vi "W7XBolo2018.vi"(1 "FPGA VI Reference In":refnum<k20>) -> (0 "FPGA VI Reference Out":refnum<k20>)   [LabVIEW 2014]
uses:
  <vilib>/Platform/TimedLoop/XDataNode/timing_clust.ctl
  <vilib>/Platform/TimedLoop/XDataNode/nitl_modes.ctl
  <vilib>/Platform/TimedLoop/XDataNode/wakeup.ctl
  <vilib>/userdefined/High Color/nirio_resource_hc.ctl
  <vilib>/DAQmx/write.llb/DAQmx Write (Analog 1D DBL 1Chan NSamp).vi
  <vilib>/FPGAPlugInAG/PCI-7813R/niLvFpga_Open_PCI-7813R.vi
  <vilib>/Utility/error.llb/Error Cluster From Error Code.vi
  <vilib>/rvi/errors/niLvFpgaAdjustHostInterfaceError.vi
  <vilib>/rvi/interface/common/niFpgaWaitOnOcc.vi
  <vilib>/DAQmx/create/channels.llb/DAQmx Create Channel (AO-Voltage-Basic).vi
  <vilib>/DAQmx/configure/timing.llb/DAQmx Timing (Sample Clock).vi
  <vilib>/DAQmx/miscellaneous.llb/DAQmx Fill In Error Info.vi
  <vilib>/httpClient/POSTBuffer.vi
  <vilib>/FPGAPlugInAG/PCI-7813R/niLvFpga_Close_PCI-7813R.vi
  <vilib>/Utility/file.llb/Read From Spreadsheet File (DBL).vi
  <vilib>/Utility/file.llb/Read From Spreadsheet File (I64).vi
  <vilib>/Platform/TimedLoop/XDataNode/XDataNode.xnode
  <vilib>/rvi/interface/nirviOpenFPGA/nirviOpenFPGA.xnode
  FPGA Bitfiles/W7XBolo2017_FPGATarget_fmain2014_9xlV3GyHFfo.lvbitx
  f_main_2014.vi
  <vilib>/rvi/interface/nirviReadWriteControl/nirviReadWriteControl.xnode
  <vilib>/rvi/interface/nirviMethod/nirviMethod.xnode
  <vilib>/rvi/interface/nirviCloseFPGA/nirviCloseFPGA.xnode
  <vilib>/Platform/TimedLoop/XDataNode/XDNodeRunTimeDep.lvlib
  <vilib>/Analysis/NI_AALBase.lvlib
  <vilib>/httpClient/LabVIEWHTTPClient.lvlib
  <resource>/objmgr/daqmx.rc
  NiFpgaLv.dll
  <vilib>/FPGAPlugInAG/PCI-7813R/niLvFpga_AcknowledgeIrq_PCI-7813R.vi
  <vilib>/FPGAPlugInAG/PCI-7813R/niLvFpga_ConfigureFifo_PCI-7813R.vi
  <vilib>/rvi/errors/niLvFpgaMergeErrorWithErrorCode.vi
panel:
  out "Time until Acqusition":dbl(slide)=4294967295.0 scale=0.0..60.0
  out "start time":i64
  out "trigger time final":i64
  out "DAQ Timer":dbl
  in  "Tab Control 7":T1(tab)
  in  "FreqSelRing":u16(ring) items=["0.8 ms", "1.6 ms", "3.2 ms", "6.4 ms", "12.8 ms", "19.2 ms"]
  in  "SecondFilter":bool=TRUE
  out "SampleTime":sgl=0.0008
  in  "global or individual DAC settings for knob":bool caption="Range?"
  in  "DAC Range Setting":u8(knob)=3 scale=0.0..3.0
  out "No. of Samples\n[TOA / Sample Rate]":u32=10000
  out "Measured Time for DAQ [ms]\n\nApprox. ~ SampleTime * Samples":u32
  in  "?":bool=TRUE
  in  "DAC settings file location":path=path "C:/LABVIEW/BLV Philipp/LABVIEW/BLV/bolo_files/dac_settings.dat"
  in  "Time of Acqusition [s]":dbl=10.0
  out "predicted time [ms] to finalize DAQ":dbl
  in  "Read Channel Selection from file":bool=TRUE
  in  "Path to channel selection file":path=path "C:/LABVIEW/BLV Philipp/LABVIEW/BLV/bolo_files/short_channel_selection.dat"
  in  "Path to kbolott and volume data file":path=path "C:/LABVIEW/BLV Philipp/LABVIEW/BLV/bolo_files/kbolott_volume_all.dat"
  in  "Read geometry from file?":bool=TRUE
  in  "Trigger Source":i32(slide)=2 scale=0.0..3.0
  in  "Set Manual Time [ns], default updated last on 06/20/2018":i64=1529501124000000000
  out "Presamples \n(If -1, then no trigger detected)":i32
  out "DAQ wait time (should be = TWT":i32=-1
  out "Countdown Time":u32
  out "Calibration Time":u32
  out "Total wait time (TWT)\nTypically 59 s":u32
  in  "Pre-start time (ms) of DAQ \nTypically set to 1000 ms":i32=1000
  in  "Fixed T-60sec before T1 = T0":i32=60000
  in  "waiting time 'til trigger\npublished by CODAC":u32=10000
  out "Number of nanoseconds with offset to 1904":i64
  out "current epoch time timestamp":timestamp
  in  "Tau00":dbl[](array[numeric])=[0.11491729291343579, 0.11716798919571741, 0.11740631364396965, 0.11663726342199245, 0.41599980468961384, 0.11981011551839264, 0.11846429840933606, 0.11867732465684001, 0.1099546558688366, 0.11157519276959196, 0.10652596659944064, 0.11187533014192738, 0.11242534122168901, 0.11250590452650158, 0.11233958629056463, 0.11088956837703348, 0.11684290859752998, 0.11711408209103276, 0.11862962903855054, 0.11574688850921441, 0.11080958640139682, 0.11308007616237671, 0.11316833203019577, 0.11732662567656041, 0.11776955995449861, 0.11488434870753593, 0.11721346913661516, 0.11723600482803162, 0.1173219143188469, 0.11486538187917118, 0.1161354905419326, 0.11580597702447244, 0.11089805083278159, 0.10965173450878267, 0.10989266890532523, 0.11049724960692761, 0.11094253276914103, 0.1112015939579455, 0.11056511595580205, 0.11125203268352817, 0.10851766683731974, 0.10665739286095859, 0.10665088457538054, 0.10647759616581123, 0.10805487600009084, 0.10533289893772232, 0.10446227511758968, 0.10416638033440741, 0.11156846805821136, 0.11129308727212155, 0.11117840263008584, 0.1102971572868625, 0.10837301568677209, 0.11586325578254852, 0.11338638335503164, 0.11266837385466463, 0.11020464539493718, 0.11718312222258088, 0.11005940383900907, 0.11074035298635442, 0.11310264754168789, 0.11428021968521139, 0.10890693978140649, 0.11304857784773828, 0.11071164775178235, 0.10899043148625223, 0.1098152132889097, 0.11071094104034687, 0.10922727710545306, 0.11026461123495493, 0.10902110264823185, 0.1063818330991493, 0.1082901421909468, 0.10855104773097228, 0.10976304069098969, 0.1092806529611063, 0.10813898027014157, 0.10856892511543396, 0.10528805150138838, 0.10996755406311447, 0.11441717863822966, 0.11512938300201939, 0.11354812708860414, 0.11170183444428032, 0.10929951535815542, 0.10880924561891742, 0.11032002393110663, 0.12233406623444484, 0.10819046523889579, 0.10676534101945172, 0.11334069041654328, 0.11395839570756812, 0.10860855876008385, 0.11000092792604536, 0.11150855742531308, 0.11072296835591808, 0.11248944715419666, 0.11109385151927784, 0.10904702395407219, 0.0, 0.11012618939531567, 0.1101228599630128, 0.10901646637252452, 0.10848342666256441, 0.1118672405375629, 0.11165093132257785, 0.11030651312297526, 0.1105637825970819, 0.10972695234743621, 0.11008183794997571, 0.10869604711918752, 0.0, 0.10947241009391531, 0.5898071300815099, 0.41732939048318163, 0.0, 0.0, 0.0, 0.0, 0.0, 0.0, 0.0, 0.5051635137410128, 0.0, 0.0, 0.0, 0.4056247218989413, 0.0, 0.11491729291343579]
  in  "Kappa00":dbl[](array[numeric])=[0.0008402794220111138, 0.0008162628511746609, 0.0008306690902202418, 0.000803901120831155, 0.0003482758920990883, 0.0008106589659042871, 0.0008016286027972057, 0.000799559666964026, 0.0008329596140242245, 0.0008550459829924856, 0.0007662506038997399, 0.0008054791716010769, 0.0008538518247154832, 0.0008293547031323884, 0.0008561853513376051, 0.0008533408283799155, 0.0008374094293251158, 0.0008246891754373999, 0.0008094405414334474, 0.0008290847564626268, 0.00020601047667132065, 0.000800173048893566, 0.0007793179002779764, 0.0007971071724399289, 0.0007885266906587188, 0.0007777314742190596, 0.000805938950941268, 0.0007876903707101731, 0.0008486502743123638, 0.0008188176160358826, 0.0008275575494250777, 0.0008021526930523769, 0.0004219866202355569, 0.0008028836567896177, 0.0007965332650444257, 0.0007657694302588966, 0.0007891955147847732, 0.0007918255330716038, 0.0007896451983246505, 0.0007639621417921391, 0.0008241807402430576, 0.0008494655305824806, 0.0008513286284044697, 0.0008584599469876866, 0.0008065529851855167, 0.0008583681445476364, 0.0008848769105909991, 0.0008824761623272339, 0.0008739299904558458, 0.0008726933272884011, 0.0008591817798513973, 0.0008546408142867519, 0.0008814192063552359, 0.000837962132357275, 0.0008754373245495078, 0.0008659455513111399, 0.000875854800823488, 0.0008145627712648352, 0.000847096348180231, 0.0008354027185001123, 0.0008988684127044384, 0.0009087972104601418, 0.000872460372055295, 0.0008865774530667089, 0.0008205858447961992, 0.0008661153610700915, 0.0008514123741077071, 0.0008674455175914637, 0.0008535020874821334, 0.0008530135268333135, 0.0008817680910658127, 0.0008857682842425993, 0.0009014333315122717, 0.0009058705470039874, 0.0009451074888355545, 0.0008658347728111954, 0.0008865415114476586, 0.0009037142514292518, 0.0009300212486309693, 0.0009201252229947723, 0.0008662494433570838, 0.0008561155107896092, 0.0008934103962644251, 0.000843038472812381, 0.0008821165464311927, 0.0008725326170488139, 0.0008607956284658778, 0.0008692253024054895, 0.0007600922149492939, 0.0007595503979645458, 0.0008808740943017723, 0.0008427393057336779, 0.0008151549367042052, 0.0008178123459529788, 0.0008143006723436752, 0.0008042217964108747, 0.0007735257506859799, 0.0007705827889143488, 0.0007855750338204015, 1.5378016423296697e-10, 0.0007777843483157151, 0.0007914940873736198, 0.0007883969825026242, 0.000818379256343944, 0.0008183032224836934, 0.0008253700992517207, 0.0008193590844345892, 0.0008108478163956726, 0.0007992276276126246, 0.0007886605041422787, 0.000781928010070813, 1.3117348375603198e-11, 0.0007692233287415738, -6.433477601629483e-12, 5.840652071940865e-11, -5.095362431956802e-12, 1.483332911600832e-10, -2.3650890104320048e-11, 2.0638470359814695e-11, -4.2942497083098924e-12, -1.609109206826474e-13, -8.281241741308274e-13, -1.484842606490482e-11, 1.312154360785075e-10, -1.3280672580076002e-10, 3.875382814091509e-11, -5.840342459280051e-12, 1.6602972107316198e-05]
  in  "RB000":dbl[](array[numeric])=[962.4177063722611, 982.55505646202, 1001.4524254455091, 1013.2686972880372, 987.9006509030032, 991.6776299499904, 1028.1941896508492, 1025.4234890548287, 979.6474971153391, 974.5100933960157, 973.0002231971498, 981.3770747072988, 943.3083319407024, 941.9659261539757, 935.9901166328577, 922.8756359883505, 1000.2356401751263, 1016.4518014388639, 1008.5518682535671, 995.9759478197891, 1393.1164953762932, 1009.4128515400009, 1004.0036749391834, 998.4245511355359, 1013.969149931135, 1006.3653804065095, 999.1527693687324, 1010.8263977028598, 907.9396854856363, 919.914547854408, 928.8836112172035, 935.6473530653229, 1831.0832629084102, 903.0974305802013, 913.186368963444, 930.0383764679839, 876.4924197978996, 886.7670713082508, 894.536808158485, 915.0431333478505, 950.9758424469715, 947.5925766523108, 943.7054707777233, 932.0275841045941, 942.1982964674207, 920.3009912512268, 906.1613034702182, 900.8719996970515, 995.3340306419007, 1002.2623248554355, 1009.982778992568, 1020.4549365978846, 985.7853875544756, 1010.0388934379409, 924.365648284157, 938.198768243208, 984.5084426613569, 1028.1136001647244, 994.3062769668693, 996.1192994757585, 934.9355121674548, 939.7126408239549, 972.6026561318754, 952.3887606547273, 984.9574148687554, 938.8738492860468, 980.1140933255242, 976.5349653385726, 992.7415178653471, 992.5396366956102, 987.4159973831593, 984.3966487516718, 977.1474302625734, 949.6506551232892, 925.9244618646749, 977.9525359780853, 965.5702842228591, 958.1238603805732, 947.99064876123, 929.4112824181327, 921.0026412584975, 923.0539958218653, 922.9112208417712, 993.6091773425921, 967.4949115866236, 971.1288101242847, 976.32752644686, 1330.674292830122, 949.3495655938384, 944.3884832069355, 931.3665988355956, 938.4573966906173, 873.9327397917785, 861.7506061462778, 853.2628755931436, 852.3451337346856, 952.8804870925069, 966.9750479771292, 968.5993925762996, 0.0, 932.9605694732488, 935.3958729949309, 938.085486227425, 937.2411392500057, 848.2825097854029, 856.1379994596109, 865.233945109098, 882.1024138917886, 890.4810243739747, 897.2026495346195, 913.1867276731607, 0.0, 917.2859168494497, 0.0, 0.0, 0.0, 0.0, 0.0, 0.0, 0.0, 0.0, 0.0, 0.0, 0.0, 0.0, 0.0, 0.0, 0.0]
  in  "Switch to fixed \nCalibration Values":bool
  in  "Clear all Values \nfrom Beginning":bool
  in  "Cancel Button":bool
  out "Actual Depth":u32=256
  out "T-Start [for Display)\nShould be -1 [s]":sgl=-1.0
  in  "Trigger No Choice\nfrom MDS+ Website\n0 for old\n1 during OP":i32
  out "ScandID read/write error, late":errorcluster
  out "ScanID":u32
  in  "Tab Control":T2(tab)
  in  "Tab Control 4":enum32{"1 to 64", "65 to 128"}(tab)
  out "Raw 33-64":T3={"Channels 33 - 40"={"tstart"=-1.0, "FPGSampleTime"=0.0007999999797903001, array8x10000[80000 elements]}, "Channels 41 - 48"={"tstart"=-1.0, "FPGSampleTime"=0.0007999999797903001, array8x10000[80000 elements]}, "Channels 49 - 56"={"tstart"=-1.0, "FPGSampleTime"=0.0007999999797903001, array8x10000[80000 elements]}, "Channels 57 - 64"={"tstart"=-1.0, "FPGSampleTime"=0.0007999999797903001, array8x10000[80000 elements]}}
  out "Raw 1-32":T4={"Channels 1- 8"={"tstart"=-1.0, "FPGSampleTime"=0.0007999999797903001, array8x10000[80000 elements]}, "Channels 9 - 16"={"tstart"=-1.0, "FPGSampleTime"=0.0007999999797903001, array8x10000[80000 elements]}, "Channels 17 - 24"={"tstart"=-1.0, "FPGSampleTime"=0.0007999999797903001, array8x10000[80000 elements]}, "Channels 25 - 32"={"tstart"=-1.0, "FPGSampleTime"=0.0007999999797903001, array8x10000[80000 elements]}}
  out "Raw 97 - 128":T5
  out "Raw 65 - 97":T6={"Channels 65 - 71"={"tstart"=-1.0, "FPGSampleTime"=0.0007999999797903001, array8x10000[80000 elements]}, "Channels 73 - 80"={"tstart"=0.0, "FPGSampleTime"=0.0, []}, "Channels 81 - 88"={"tstart"=0.0, "FPGSampleTime"=0.0, []}, "Channels 89- 96"={"tstart"=0.0, "FPGSampleTime"=0.0, []}}
  out "RawArray":sgl[][](array[numeric])
  in  "Tab Control 6":enum32{"1 to 64", "65 to 128"}(tab)=enum."65 to 128"
  out "Pow 33-64":T3
  out "Pow 1-32":T4={"Channels 1- 8"={"tstart"=-1.0, "FPGSampleTime"=0.0007999999797903001, array8x10000[80000 elements]}, "Channels 9 - 16"={"tstart"=-1.0, "FPGSampleTime"=0.0007999999797903001, array8x10000[80000 elements]}, "Channels 17 - 24"={"tstart"=0.0, "FPGSampleTime"=0.0, []}, "Channels 25 - 32"={"tstart"=0.0, "FPGSampleTime"=0.0, []}}
  out "Pow 97 - 128":T5
  out "Pow 65 - 96":T6={"Channels 65 - 71"={"tstart"=-1.0, "FPGSampleTime"=0.0007999999797903001, array8x10000[80000 elements]}, "Channels 73 - 80"={"tstart"=0.0, "FPGSampleTime"=0.0, []}, "Channels 81 - 88"={"tstart"=0.0, "FPGSampleTime"=0.0, []}, "Channels 89- 96"={"tstart"=0.0, "FPGSampleTime"=0.0, []}}
  out "PowerArray":sgl[][](array[numeric])
  out "real time P_rad plot":cluster{i32, "element":dbl, "element":dbl}[](graph)
  out "Channel Selection\nfrom input?":bool
  out "DAC settings":i64[](array[numeric])=[3, 3, 3, 3, 3, 3, 3, 3, 3, 3, 3, 3, 3, 3, 3, 3, 3, 3, 3, 3, 3, 3, 3, 3, 3, 3, 3, 3, 3, 3, 3, 3, 3, 3, 3, 3, 3, 3, 3, 3, 3, 3, 3, 3, 3, 3, 3, 3, 3, 3, 3, 3, 3, 3, 3, 3, 3, 3, 3, 3, 3, 3, 3, 3, 3, 3, 3, 3, 3, 3, 3, 3, 3, 3, 3, 3, 3, 3, 3, 3, 3, 3, 3, 3, 3, 3, 3, 3, 3, 3, 3, 3, 3, 3, 3, 3, 3, 3, 3, 3, 3, 3, 3, 3, 3, 3, 3, 3, 3, 3, 3, 3, 3, 3, 3, 3, 3, 3, 3, 3, 3, 3, 3, 3, 3, 3, 0, 0]
  out "size(s)":i32
  out "Take file for DAC?":bool
  out "full DAC\nfile input":i64[][](array[numeric])=[[3], [3], [3], [3], [3], [3], [3], [3], [3], [3], [3], [3], [3], [3], [3], [3], [3], [3], [3], [3], [3], [3], [3], [3], [3], [3], [3], [3], [3], [3], [3], [3], [3], [3], [3], [3], [3], [3], [3], [3], [3], [3], [3], [3], [3], [3], [3], [3], [3], [3], [3], [3], [3], [3], [3], [3], [3], [3], [3], [3], [3], [3], [3], [3], [3], [3], [3], [3], [3], [3], [3], [3], [3], [3], [3], [3], [3], [3], [3], [3], [3], [3], [3], [3], [3], [3], [3], [3], [3], [3], [3], [3], [3], [3], [3], [3], [3], [3], [3], [3], [3], [3], [3], [3], [3], [3], [3], [3], [3], [3], [3], [3], [3], [3], [3], [3], [3], [3], [3], [3], [3], [3], [3], [3], [3], [3]]
  in  "input DAC settings":i64[](array[numeric])=[3, 3, 3, 3, 3, 3, 3, 3, 3, 3, 3, 3, 3, 3, 3, 3, 3, 3, 3, 3, 3, 3, 3, 3, 3, 3, 3, 3, 3, 3, 3, 3, 3, 3, 3, 3, 3, 3, 3, 3, 3, 3, 3, 3, 3, 3, 3, 3, 3, 3, 3, 3, 3, 3, 3, 3, 3, 3, 3, 3, 3, 3, 3, 3, 3, 3, 3, 3, 3, 3, 3, 3, 3, 3, 3, 3, 3, 3, 3, 3, 3, 3, 3, 3, 3, 3, 3, 3, 3, 3, 3, 3, 3, 3, 3, 3, 3, 3, 3, 3, 3, 3, 3, 3, 3, 3, 3, 3, 3, 3, 3, 3, 3, 3, 3, 3, 3, 3, 3, 3, 3, 3, 3, 3, 3, 3, 0, 0]
  out "Take Input for DAC?":bool
  out "kbolott_and_volume":dbl[][](array[numeric])
  out "final channel\nselection size":i32
  out "final channel selection":i64[][](array[numeric])=[[0], [1], [2], [3], [4], [5], [6], [7], [8], [9], [10], [11], [12], [13], [14], [15], [16], [17], [18], [19], [20], [21], [22], [23], [24], [25], [26], [27], [28], [29], [30], [31]]
  in  "channel selection input":i32[][](array[numeric])=[[1]]
  out "file import":i64[][](array[numeric])
  in  "maximum voltage @ 10MW\nP_rad estimate":dbl=10.0 format="%#_13g"
  out "number of samples per iteration":dbl
  out "number of samples written on channel":u32
  in  "rate of voltage sampling":dbl=100000.0 format="%#_13g"
  in  "RegenMode":i32(ring)=10158 items=["Allow Regeneration"=10097, "Do Not Allow Regeneration"=10158]
  in  "sample mode":i32(ring)=10123 items=["Finite Samples"=10178, "Continuous Samples"=10123, "Hardware Timed Single Point"=12522]
  in  "Stop Voltage Output":bool
  out "current P_rad sample [MW]":dbl format="%#_13g"
  out "final P_rad":dbl[](array[numeric])
  out "av power array":dbl[](array[numeric])
  out "P_rad analog output error source":string
  in  "DAQmx Physical Channel\nP_rad estimate":tag="Dev1/ao0"
  out "nominator":dbl
  out "number of samples \nwritten per channel":u32
  in  "selected channel for output via second analog channel":i32
  in  "estimated floating voltage":dbl format="%#_13g"
  out "estimated voltage @ 10 MW":dbl
  out "voltage factor":dbl
  in  "DAQmx Physical Channel\nsingle channel":tag="Dev1/ao1"
  in  "maximum voltage @ 10MW single channel":dbl=10.0 format="%#_13g"
  out "single channel output error source":string
  out "current single channel voltage":dbl format="%#_13g"
  out "single channel voltage array":dbl[](array[numeric])
  out "P_rad output\nvoltage":dbl
  out "single channel voltage output [MW]":dbl
  in  "voltage fac":dbl=10000.0
  out "RangeIndex":u8[](array[numeric])
  out "DACbits 2":u16[](array[numeric])
  out "x*2^n":sgl[](array[numeric])
  in  "Tab Control 2":T7(tab)
  out "Offset 1-32":T4
  out "Offset 33-64":T3
  out "Offset 65 - 96":T6
  out "Offset 97 - 128":T5
  out "Mean (mV)":dbl[](array[numeric]) format="%10.6f"
  out "Peak to Peak \n      (microV)":dbl[](array[numeric]) format="%10.6f"
  out "StandardDeviation\n        (microV)":dbl[](array[numeric]) format="%10.7f"
  out "Offset (V)":dbl[](array[numeric])
  out "RefStatus 65-96":bool[](array[boolean])
  out "RefStatus 33-64":bool[](array[boolean])
  out "RefStatus 1-32":bool[](array[boolean])
  out "RefStatus 97-128":bool[](array[boolean])
  out "MessStatus 1-32":bool[](array[boolean])
  out "MessStatus 33-64":bool[](array[boolean])
  out "MessStatus 97-128":bool[](array[boolean])
  out "MessStatus 65-96":bool[](array[boolean])
  in  "Tab Control 5":T8(tab)
  out "MessCal 17-32":T9
  out "MessCal 1-16":T10
  out "MessCal 49 - 64":T11
  out "MessCal 33 - 49":T12
  out "MessCal 81 - 96":T13
  out "MessCal 65 - 80":T14
  out "MessCal 113 - 128":T15
  out "MessCal 97 - 112":T16
  out "TauM":dbl[](array[numeric]) format="%10.4f"
  out "KappaM":dbl[](array[numeric]) format="%10.4e"
  out "RMESS":dbl[](array[numeric])
  out "RawScal":dbl[](array[numeric])
  out "ScalPower":dbl[](array[numeric])
  out "Tau":dbl[](array[numeric])
  out "F_ch":dbl[](array[numeric])
  out "tau_fact":dbl[](array[numeric])
  in  "Tab Control 3":T8(tab)=enum."97 to 128"
  out "RefCal 17-32":T9
  out "RefCal 1-16":T10
  out "RefCal 49 - 64":T11
  out "RefCal 33 - 48":T12
  out "RefCal 65 - 80":T14
  out "RefCal 81 - 96":T13
  out "RefCal 113 - 128":T15
  out "RefCal 97 - 112":T16
  out "TauR":dbl[](array[numeric]) caption="TauM" format="%10.4f"
  out "KappaR":dbl[](array[numeric]) format="%10.4e"
  out "RREF":dbl[](array[numeric])
  out "BoloCalibRefFoilFit data error":errorcluster
  out "BoloCalibRefFoilCurrent data error":errorcluster
  out "fpga_reference\nOpen error out":errorcluster
  out "Timed Out 2":bool
  out "Fehler":bool
  out "Fehler READ U+P":bool
  out "FilterTimeOut":bool
  out "result":bool
  out "error out Cal":errorcluster
  out "headers chanDesc":string="HTTP/1.1 201 Created\r\nServer: Apache-Coyote/1.1\r\nLocation: http://archive-webapi.ipp-hgw.mpg.de/Test/raw/W7X/QSB_Bolometry/File_PARLOG/\r\nContent-Type: text/plain\r\nTransfer-Encoding: chunked\r\nDate: Wed, 15 Jul 2015 13:52:20 GMT\r\n\r\n"
  out "body chanDesc":string="Test/raw/W7X/QSB_Bolometry/File_PARLOG/ created."
  out "parms error out":errorcluster
  out "error after hReadDMA":errorcluster
  out "ScandID read/write error, early":errorcluster
  out "ScanID 2":u32
  out "BoloCalibMeasFoilFit data error":errorcluster
  out "BoloSignal data error":errorcluster
  out "BoloCalibMeasFoilCurrent\ndata error":errorcluster
  out "rRes parlog error":errorcluster
  out "rKappa parlog error":errorcluster
  out "mTau parlog error":errorcluster
  out "offset parlog error":errorcluster
  out "mRes parlog error":errorcluster
  out "mKappa parlog error":errorcluster
  out "rTau parlog error":errorcluster
  out "loop error":errorcluster
  out "sampling error":errorcluster
  out "voltage sampling error":T17
  in  "SubVI Test\nwith RAND array and\ntime measurement":bool
  out "random array sub":dbl[](array[numeric])
  out "random array main":dbl[](array[numeric])
  out "sample array":i32[](array[numeric])
  out "subvi cycle #":dbl
  out "subvi timing":dbl
  out "pick-up cycle":i32
  out "total\ntime":dbl
  out "timing average":dbl format="%.2f"
  out "rand array sub display":dbl[](array[numeric])
  out "rand plot sub":cluster{i32, "element":dbl}[](graph)
  out "cycle #":i32
  out "rand plot main":cluster{i32, "element":dbl}[](graph)
  out "empty write array":dbl[](array[numeric])
  out "Nsample array":i32[](array[numeric])
  in  "stop":bool
  out "Acquired Samples:":u32(slide)=4294967295 scale=-1.0..10000.0
  out "state":string="Wait for Start"
  # "largest offset ~ 40 mV\n-- 40 mV should work --\n-- 80 mV safe setting --"
  # "Sample Rate Settings"
  # "FilterSelection"
  # "put time stamp of now as\nPOSIX time in [ns] as trigger"
  # "Set manual time\n[epoch time, ns since 01.01.1970]"
  # "Get last trigger from \nhttp://sv-coda-wsvc-3/last_trigger"
  # "Get UTC Time not working"
  # "WENDELSTEIN - 7-X Bolometer DAQ System [mail at: pih@ipp.mpg.de]"
  # "ver 2018"
  # "If individual Range DAC Setting is selected, \nthe gain Range is loaded from following file:"
  # "DAC Range shown for check:"
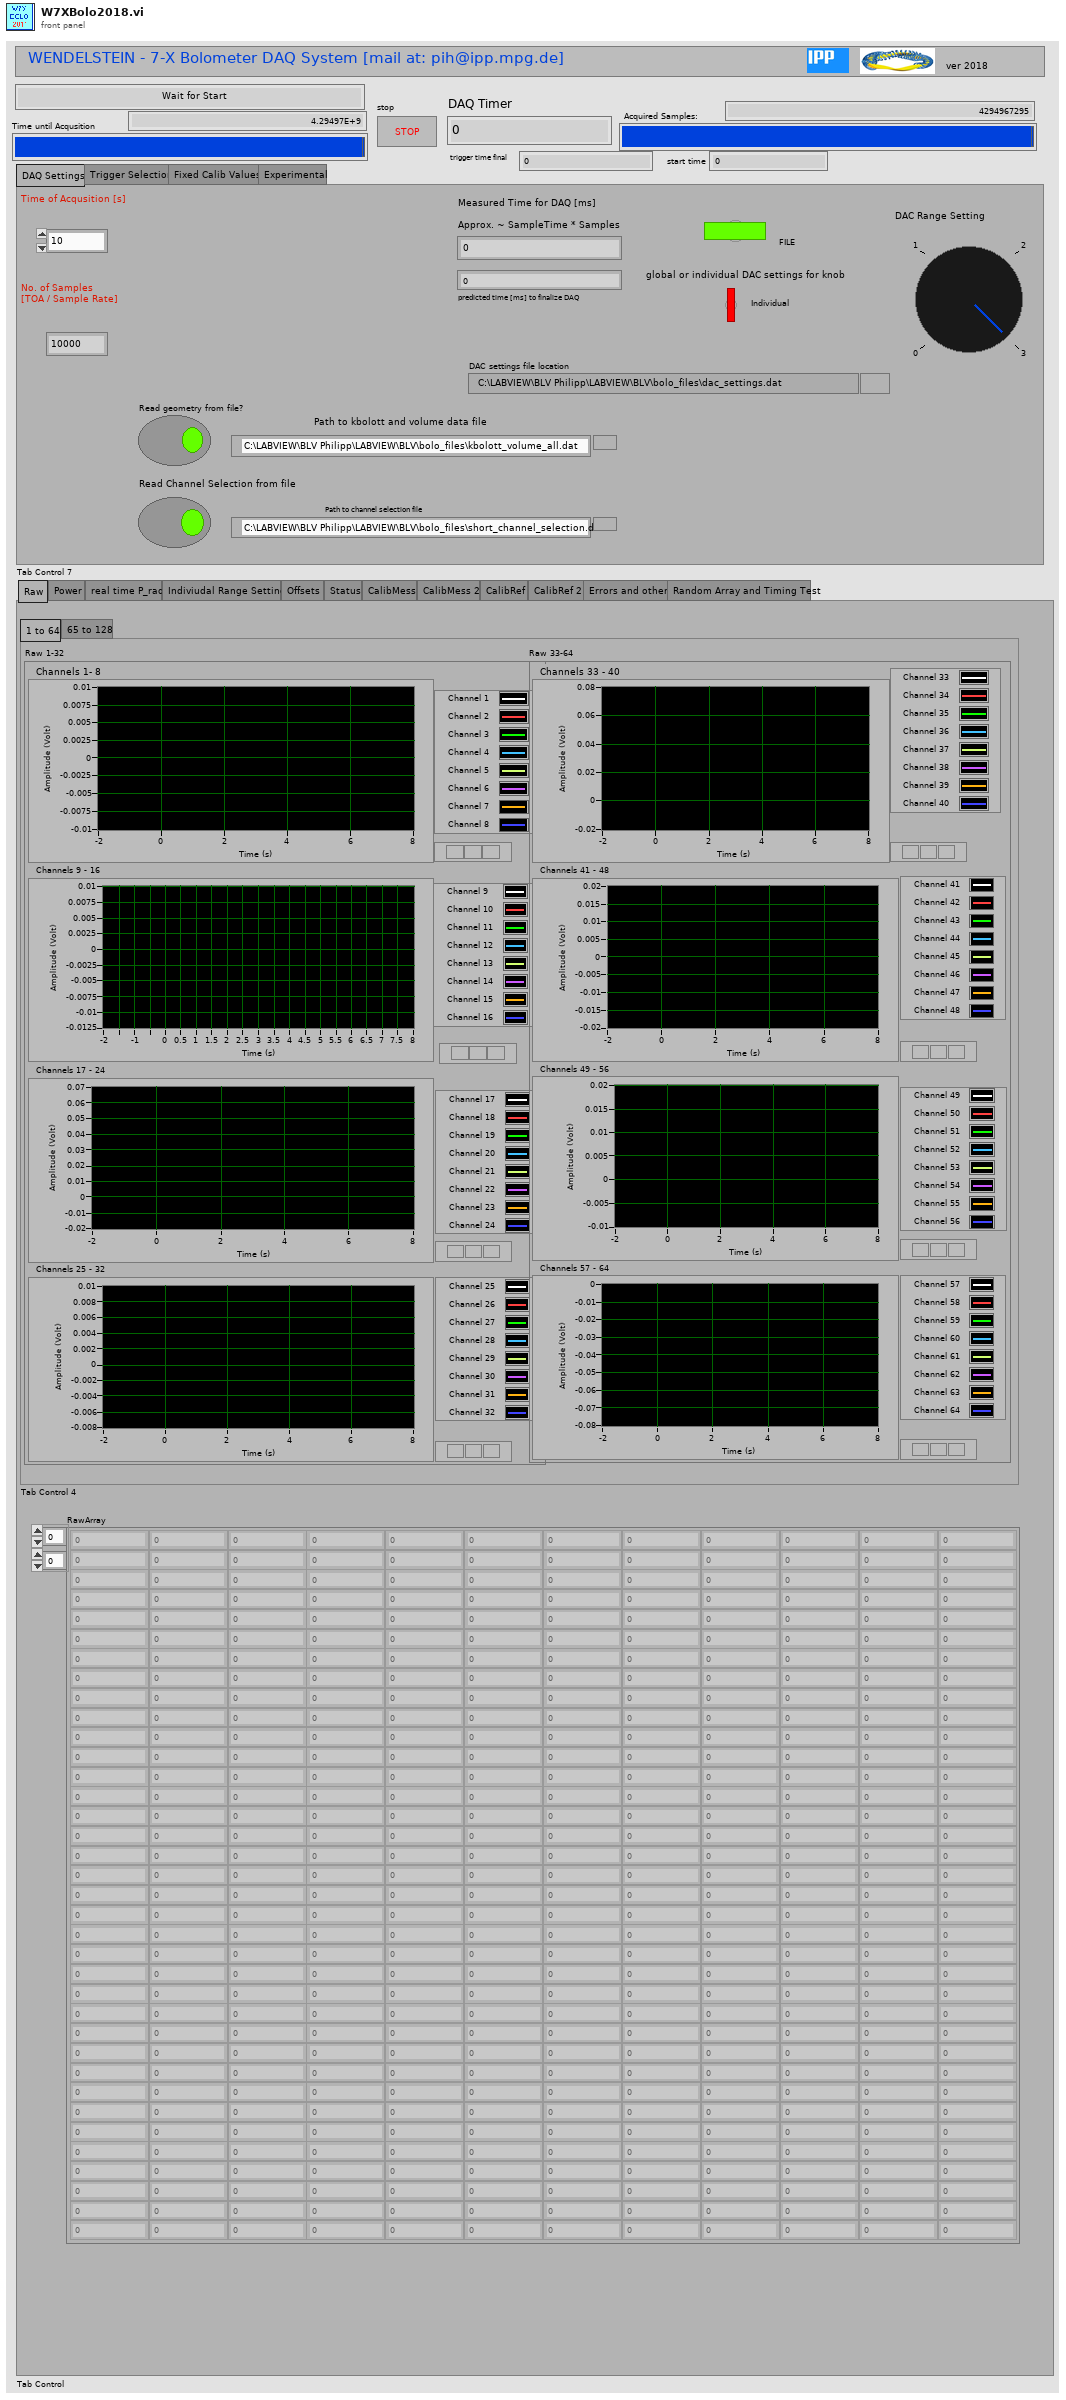
[diagram p1: front panel]
types:
  T1 = enum32{"DAQ Settings", "Trigger Selection", "Fixed Calib Values", "Experimental"}
  T2 = enum32{"Raw", "Power", "real time P_rad", "Indiviudal Range Settings", "Offsets", "Status", "CalibMess", "CalibMess 2", "CalibRef", "CalibRef 2", "Errors and others", "Random Array and Timing Test"}
  T3 = cluster{"Channels 33 - 40":cluster{"tstart":dbl, "FPGSampleTime":dbl, dbl[][]}, "Channels 41 - 48":cluster{"tstart":dbl, "FPGSampleTime":dbl, dbl[][]}, "Channels 49 - 56":cluster{"tstart":dbl, "FPGSampleTime":dbl, dbl[][]}, "Channels 57 - 64":cluster{"tstart":dbl, "FPGSampleTime":dbl, dbl[][]}}
  T4 = cluster{"Channels 1- 8":cluster{"tstart":dbl, "FPGSampleTime":dbl, dbl[][]}, "Channels 9 - 16":cluster{"tstart":dbl, "FPGSampleTime":dbl, dbl[][]}, "Channels 17 - 24":cluster{"tstart":dbl, "FPGSampleTime":dbl, dbl[][]}, "Channels 25 - 32":cluster{"tstart":dbl, "FPGSampleTime":dbl, dbl[][]}}
  T5 = cluster{"Channels 97 - 104":cluster{"tstart":dbl, "FPGSampleTime":dbl, dbl[][]}, "Channels 105 - 112":cluster{"tstart":dbl, "FPGSampleTime":dbl, dbl[][]}, "Channels 113 - 120":cluster{"tstart":dbl, "FPGSampleTime":dbl, dbl[][]}, "Channels 121 - 128":cluster{"tstart":dbl, "FPGSampleTime":dbl, dbl[][]}}
  T6 = cluster{"Channels 65 - 71":cluster{"tstart":dbl, "FPGSampleTime":dbl, dbl[][]}, "Channels 73 - 80":cluster{"tstart":dbl, "FPGSampleTime":dbl, dbl[][]}, "Channels 81 - 88":cluster{"tstart":dbl, "FPGSampleTime":dbl, dbl[][]}, "Channels 89- 96":cluster{"tstart":dbl, "FPGSampleTime":dbl, dbl[][]}}
  T7 = enum32{"1 to 32", "33 to 64", "65 to 96", "97 to128"}
  T8 = enum32{"1 to 32", "33 to 64", "65 to 96", "97 to 128"}
  T9 = cluster{"Channels 17 - 20":cluster{"tstart":sgl, "dt":sgl, "OutArray":dbl[][]}, "Channels 21 - 24":cluster{"tstart":sgl, "dt":sgl, "OutArray":dbl[][]}, "Channels 25 - 28":cluster{"tstart":sgl, "dt":sgl, "OutArray":dbl[][]}, "Channels 29 - 32":cluster{"tstart":sgl, "dt":sgl, "OutArray":dbl[][]}}
  T10 = cluster{"Channels 1- 4":cluster{"tstart":sgl, "dt":sgl, "OutArray":dbl[][]}, "Channels 5 - 8":cluster{"tstart":sgl, "dt":sgl, "OutArray":dbl[][]}, "Channels 9 - 12":cluster{"tstart":sgl, "dt":sgl, "OutArray":dbl[][]}, "Channels 13 - 16":cluster{"tstart":sgl, "dt":sgl, "OutArray":dbl[][]}}
  T11 = cluster{"Channels 49 - 52":cluster{"tstart":sgl, "dt":sgl, "OutArray":dbl[][]}, "Channels 53 - 56":cluster{"tstart":sgl, "dt":sgl, "OutArray":dbl[][]}, "Channels 57 - 60":cluster{"tstart":sgl, "dt":sgl, "OutArray":dbl[][]}, "Channels 61 - 64":cluster{"tstart":sgl, "dt":sgl, "OutArray":dbl[][]}}
  T12 = cluster{"Channels 33 - 36":cluster{"tstart":sgl, "dt":sgl, "OutArray":dbl[][]}, "Channels 37 - 40":cluster{"tstart":sgl, "dt":sgl, "OutArray":dbl[][]}, "Channels 41 - 44":cluster{"tstart":sgl, "dt":sgl, "OutArray":dbl[][]}, "Channels 45 - 48":cluster{"tstart":sgl, "dt":sgl, "OutArray":dbl[][]}}
  T13 = cluster{"Channels 81 - 84":cluster{"tstart":sgl, "dt":sgl, "OutArray":dbl[][]}, "Channels 85 - 88":cluster{"tstart":sgl, "dt":sgl, "OutArray":dbl[][]}, "Channels 89 - 92":cluster{"tstart":sgl, "dt":sgl, "OutArray":dbl[][]}, "Channels 93 - 96":cluster{"tstart":sgl, "dt":sgl, "OutArray":dbl[][]}}
  T14 = cluster{"Channels 65 - 68":cluster{"tstart":sgl, "dt":sgl, "OutArray":dbl[][]}, "Channels 69 - 72":cluster{"tstart":sgl, "dt":sgl, "OutArray":dbl[][]}, "Channels 73 - 76":cluster{"tstart":sgl, "dt":sgl, "OutArray":dbl[][]}, "Channels 77 - 80":cluster{"tstart":sgl, "dt":sgl, "OutArray":dbl[][]}}
  T15 = cluster{"Channels 113 - 116":cluster{"tstart":sgl, "dt":sgl, "OutArray":dbl[][]}, "Channels 117 - 120":cluster{"tstart":sgl, "dt":sgl, "OutArray":dbl[][]}, "Channels 121 - 124":cluster{"tstart":sgl, "dt":sgl, "OutArray":dbl[][]}, "Channels 125 - 128":cluster{"tstart":sgl, "dt":sgl, "OutArray":dbl[][]}}
  T16 = cluster{"Channels 97 - 100":cluster{"tstart":sgl, "dt":sgl, "OutArray":dbl[][]}, "Channels 101 - 104":cluster{"tstart":sgl, "dt":sgl, "OutArray":dbl[][]}, "Channels 104 - 108":cluster{"tstart":sgl, "dt":sgl, "OutArray":dbl[][]}, "Channels 109 - 112":cluster{"tstart":sgl, "dt":sgl, "OutArray":dbl[][]}}
  T17 = cluster{"error out":errorcluster, "error out":errorcluster}
  T18 = cluster{"Nchannel":i16, "ADCbits":i16, "BridgeVoltage (V)":sgl, "ExptSampleFrequency (Hz)":sgl, "CalibSampleFrequency (Hz)":sgl, "CalStep1 (V)":string, "CalStep2 (V)":string, "detector":string}[]
  T19 = cluster{"chanDescs":cluster{"name":string, "active":i32}[]}[]
  T20 = cluster{"tstart":sgl, "dt":sgl, "OutArray":dbl[][]}
  T21 = cluster{"Channels 9 - 12":cluster{"tstart":sgl, "dt":sgl, "OutArray":dbl[][]}, "Channels 9 - 12":cluster{"tstart":sgl, "dt":sgl, "OutArray":dbl[][]}, "Channels 9 - 12":cluster{"tstart":sgl, "dt":sgl, "OutArray":dbl[][]}, "Channels 9 - 12":cluster{"tstart":sgl, "dt":sgl, "OutArray":dbl[][]}}
  T22 = typedef "nirio_resource_hc.ctl" = tag
  T23 = typedef "XDNodeRunTimeDep.lvlib/timing_clust.ctl" = cluster{"Expected End [f-1]":u64, "Actual End [f-1]":u64, "Finished Late? [f-1]":bool, "Expected End [i-1]":u64, "Actual End [i-1]":u64, "Finished Late? [i-1]":bool, "Expected Start [i]":u64, "Actual Start [i]":u64, "Expected Start [f]":u64, "Actual Start [f]":u64, "Source Name":string, "Structure Name":string, "Period":i64, "Deadline":i64, "Offset":i64, "Start":i64, "Priority":i32, "Timeout":i32, "Mode":T24, "Wakeup Reason":T25, "Error":errorcluster, "Source Type":string, "Secondary Source Type":string, "Global End Time":u64, "Global Start Time":u64, "Frame Duration":u64, "Iteration Duration":u64, "Assigned CPU":i32, "I/O Scan Engine Mode":u32}
  T24 = typedef "XDNodeRunTimeDep.lvlib/nitl_modes.ctl" = enum32{"No Change", "Process missed periods, maintain original phase", "Discard missed periods, maintain original phase", "Process missed periods, ignore original phase", "Discard missed periods, ignore original phase"}
  T25 = typedef "XDNodeRunTimeDep.lvlib/wakeup.ctl" = enum32{"Normal", "Aborted", "Asynchronous wakeup", "Timing source error", "Timed loop error", "Timeout"}
  T26 = cluster{"Channels 33 - 40":cluster{"tstart":dbl, "FPGSampleTime":dbl, dbl[][]}, "Channels 41 - 48":cluster{"tstart":dbl, "FPGSampleTime":dbl, dbl[][]}, "Channels 49 - 56":cluster{"tstart":dbl, "FPGSampleTime":dbl, dbl[][]}, "Channels 57 - 58":cluster{"tstart":dbl, "FPGSampleTime":dbl, dbl[][]}}
  T27 = cluster{"Channels 1- 8":cluster{"tstart":sgl, "dt":sgl, "OutArray":dbl[][]}, "Channels 9 - 16":cluster{"tstart":sgl, "dt":sgl, "OutArray":dbl[][]}, "Channels 17 - 24":cluster{"tstart":sgl, "dt":sgl, "OutArray":dbl[][]}, "Channels 25 - 32":cluster{"tstart":sgl, "dt":sgl, "OutArray":dbl[][]}}
  T28 = cluster{"Channels 33 - 40":cluster{"tstart":sgl, "dt":sgl, "OutArray":dbl[][]}, "Channels 41 - 48":cluster{"tstart":sgl, "dt":sgl, "OutArray":dbl[][]}, "Channels 49 - 56":cluster{"tstart":sgl, "dt":sgl, "OutArray":dbl[][]}, "Channels 57 - 58":cluster{"tstart":sgl, "dt":sgl, "OutArray":dbl[][]}}
  T29 = typedef "LabVIEWHTTPClient.lvlib/ClientHandle.ctl" = refnum<k1>
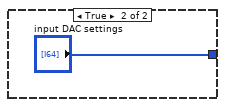
[diagram p4: hidden frame]
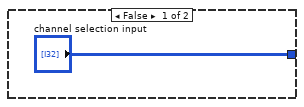
[diagram p6: hidden frame]
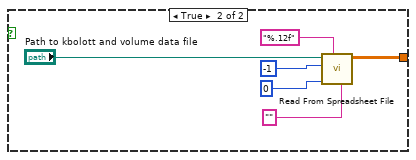
[diagram p8: hidden frame]
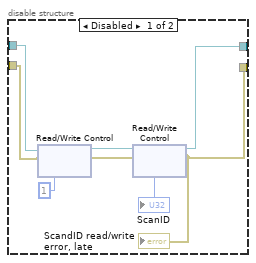
[diagram p15: hidden frame]
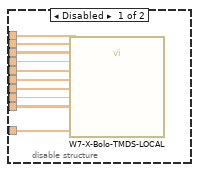
[diagram p18: hidden frame]
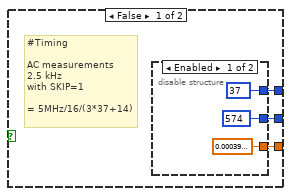
[diagram p19: hidden frame]
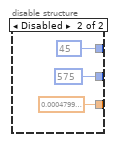
[diagram p20: hidden frame]
diagram:
  w28 = i64 -1  # Time Array needs to be positive!
  w47 = i64 -1000000000  # Ns per Sec
  w83 = 1 ("sampleCount")
  w84 = 1 ("sampleCount")
  w87 = "s"  # Unit
  w108 = "V"  # Unit
  w112 = "A"  # Unit
  w24 = "A"  # Unit
  w116 = "A"  # Unit
  w123 = 1 ("sampleCount")
  w125 = 1 ("sampleCount")
  w127 = 1 ("sampleCount")
  w82 = 1 ("sampleCount")
  w53 = 1 ("sampleCount")
  w133 = "Float"  # datatype
  w103 = "mV"  # Unit
  w105 = "Offset"  # label
  w139 = "Float"  # datatype
  w100 = "W"  # Unit
  w102 = "RKappa"  # label
  w141 = "Float"  # datatype
  w97 = "Ohms"  # Unit
  w99 = "RRes"  # label
  w143 = "Float"  # datatype
  w94 = "s"  # Unit
  w96 = "RTau"  # label
  w145 = "Float"  # datatype
  w91 = "W"  # Unit
  w93 = "MKappa"  # label
  w147 = "Float"  # datatype
  w90 = "Ohms"  # Unit
  w89 = "MRes"  # label
  w149 = "Float"  # datatype
  w86 = "MTau"  # label
  w54 = 10000 ("dimension size")
  w157 = 10000 ("sampleCount")
  w159 = "Float"  # datatype
  w118 = "A"  # Unit
  w120 = "BoloCalibRefFoilFit"  # label
  w160 = 10000 ("sampleCount")
  w162 = "Float"  # datatype
  w114 = "BoloCalibRefFoilCurrent"  # label
  w163 = 10000 ("sampleCount")
  w165 = "Float"  # datatype
  w23 = "BoloCalibMeasFoilFit"  # label
  w166 = 10000 ("sampleCount")
  w168 = "Float"  # datatype
  w110 = "BoloCalibMeasFoilCurrent"  # label
  w169 = "Float"  # datatype
  w107 = "BoloSignal"  # label
  # "Negative Sample Time [ns]"
  # "Time array for Bolo Signal"
  # "No of Samples DAQ"
  # "Time array for Bolo Signal"
  # "+ wait Time"
  # "-800000ns for 0.8ms"
  # "Negative Sample Time [ns]"
  # "Here Changed Names"
  # "Time Stamp for JSON Files"
  # "Sample rate for Calibration Arrays\n should be hardwired to calirbation settings"
  # "Sample Rate in [ns]"
  # "Calculated Start Time [ns]"
  # "NSample"
  # "10000"
  # "Initialize Array:\nDimesions Size = NSamples"
  # "Pulselength fixed for 0.4ms sample time and 10000 samples"
  # "NSamples * SampleTime = PulseLength"
  # "Data here is incorrect as well=!"
  # "Sample Time [s]\ncalculated to \nSample Time [ns]"
  # "Creating virtual Time Stamp\nfor Shot and for Calibration (Hardwired to 10000 samples)\nShot is depending on set sample rate"
  # "Index von dem Sample\nals der Trigger empfangen wurde"
  # "T1 Trigger\nkommt hier"
  # "A=> Internal full scale calibration\n8=> Internal zero scale calibration\nC=> System Zero scale Calibration\n2=> Continuous conversion\n\n5V reference\n80 mV scale\nChannel 1 input (voltage at bridge)\nMaster clock disable\n\np.15 7730 manual"
  # "AC 1.25 kHz Frequenz\nSKIP=0"
  n1 = call <vilib>:"High Resolution Relative Seconds.vi"() -> ("relative seconds"=w15:dbl)
  n2 = flat-sequence {
    tunnel: [w226] -> w72
    tunnel: ["FPGA VI Reference In"] -> w75
    tunnel: [w227] -> w16
    tunnel: w72 -> [w227]
    frame #0 {
      n3 = Tick Count (ms)() -> (millisecond timer value=w226:u32)
    }
    frame #1 {
      n4 = case shown="True" "Clear all Values \nfrom Beginning" {
        frame False {
        }
        frame True {
          n5 = flat-sequence {
            frame #0 {
              w232 = bool[] [] ("MessStatus 1-32")
              w231 = dbl[] [] ("Kappa00")
              w234 = T20 {"tstart"=0.0, "dt"=0.0, "OutArray"=[]} ("Channels 9 - 12")
              # "Clear Graphs"
              n6 = local write "RREF"(w231) -> ()
              n7 = local write "Kappa00"(w231) -> ()
              n8 = local write "TauR"(w231) -> ()
              n9 = local write "Tau00"(w231) -> ()
              n10 = local write "RB000"(w231) -> ()
              n11 = local write "RefStatus 97-128"(w232) -> ()
              n12 = local write "RefStatus 1-32"(w232) -> ()
              n13 = local write "RefStatus 33-64"(w232) -> ()
              n14 = local write "RefStatus 65-96"(w232) -> ()
              n15 = local write "KappaR"(w231) -> ()
              n16 = local write "RMESS"(w231) -> ()
              n17 = local write "MessStatus 1-32"(w232) -> ()
              n18 = local write "MessStatus 33-64"(w232) -> ()
              n19 = local write "MessStatus 65-96"(w232) -> ()
              n20 = local write "MessStatus 97-128"(w232) -> ()
              n21 = local write "KappaM"(w231) -> ()
              n22 = local write "DACbits 2"(w231) -> ()
              n23 = local write "TauM"(w231) -> ()
              n24 = Bundle("Channels 9 - 12"=w234, "Channels 9 - 12"=w234, "Channels 9 - 12"=w234, "Channels 9 - 12"=w234) -> (w233:T21)  [unwired: 1 in]
              n25 = local write "Raw 1-32"(w233) -> ()
              n26 = local write "Raw 33-64"(w233) -> ()
              n27 = local write "Pow 1-32"(w233) -> ()
              n28 = local write "Pow 33-64"(w233) -> ()
              n29 = local write "RangeIndex"(w231) -> ()
              n30 = local write "Mean (mV)"(w231) -> ()
              n31 = local write "Peak to Peak \n      (microV)"(w231) -> ()
              n32 = local write "StandardDeviation\n        (microV)"(w231) -> ()
              n33 = local write "Acquired Samples:"(0) -> ()
              n34 = local write "Raw 65 - 97"(w233) -> ()
              n35 = local write "Raw 97 - 128"(w233) -> ()
              n36 = local write "Offset 1-32"(w233) -> ()
              n37 = local write "Offset 33-64"(w233) -> ()
              n38 = local write "Offset 65 - 96"(w233) -> ()
              n39 = local write "Offset 97 - 128"(w233) -> ()
              n40 = local write "RefCal 1-16"(w233) -> ()
              n41 = local write "RefCal 113 - 128"(w233) -> ()
              n42 = local write "RefCal 17-32"(w233) -> ()
              n43 = local write "RefCal 33 - 48"(w233) -> ()
              n44 = local write "RefCal 49 - 64"(w233) -> ()
              n45 = local write "RefCal 65 - 80"(w233) -> ()
              n46 = local write "RefCal 81 - 96"(w233) -> ()
              n47 = local write "RefCal 97 - 112"(w233) -> ()
              n48 = local write "Pow 65 - 96"(w233) -> ()
              n49 = local write "Pow 97 - 128"(w233) -> ()
              n50 = local write "MessCal 1-16"(w233) -> ()
              n51 = local write "MessCal 113 - 128"(w233) -> ()
              n52 = local write "MessCal 17-32"(w233) -> ()
              n53 = local write "MessCal 33 - 49"(w233) -> ()
              n54 = local write "MessCal 49 - 64"(w233) -> ()
              n55 = local write "MessCal 65 - 80"(w233) -> ()
              n56 = local write "MessCal 81 - 96"(w233) -> ()
              n57 = local write "MessCal 97 - 112"(w233) -> ()
            }
          }
        }
      }
    }
  }
  n58 = disable-structure shown="Disabled" {
    frame Disabled {
      n59 = case shown="True" "SubVI Test\nwith RAND array and\ntime measurement" {
        frame False {
        }
        frame True {
          n60 = flat-sequence {
            tunnel: [w240] -> w237
            tunnel: [w239] -> w236
            tunnel: w237 -> [w255]
            tunnel: w236 -> [w249]
            frame #0 {
              w239 = 1000 ("x")
              n61 = Initialize Array(0, w239) -> (w244:i32[])
              n62 = for {
                N: w239 -> [_]
                shift-right: [w245] -> w240
                shift-left: w244 -> [w247]
                i -> [w246]
                n63 = Replace Array Subset(array=w247, new element=w246, index=w246) -> (w245:i32[])
              }
              "sample array" <- w240
              n64 = local write "state"("pre-occupying test arrays" ("state")) -> ()
              n65 = Initialize Array(0.0 ("element"), w239) -> (w238:dbl[])
              "random array main" <- w238
              "random array sub" <- w238
              n66 = local write "random array main"(w238) -> ()
              n67 = local write "random array sub"(w238) -> ()
            }
            frame #1 {
              # "testing for array output"
              n68 = call <vilib>:"High Resolution Relative Seconds.vi"() -> ("relative seconds"=w251:dbl)
              n69 = control-ref of="rand array sub display"() -> (w253:refnum<vi>)
              n70 = local read "No. of Samples\n[TOA / Sample Rate]"() -> (w248:u32)
              n71 = for {
                N: w248 -> [_]
                i -> [w261]
                n72 = local read "av power array"() -> (w265:dbl[])
                n73 = local read "final P_rad"() -> (w262:dbl[])
                n74 = Random Number (0-1)() -> (number: 0 to 1=w264:dbl)
                n75 = Replace Array Subset(array=w265, new element=w264, index=w261) -> (w263:dbl[])
                n76 = Random Number (0-1)() -> (number: 0 to 1=w260:dbl)
                n77 = Replace Array Subset(array=w262, new element=w260, index=w261) -> (w259:dbl[])
                n78 = local write "av power array"(w263) -> ()
                n79 = local write "final P_rad"(w259) -> ()
                n80 = Wait Until Next ms Multiple(millisecond multiple=u32 50) -> ()  [unwired: 1 out]
              }
              n81 = control-ref of="subvi cycle #"() -> (w250:refnum<vi>)
              n82 = control-ref of="subvi timing"() -> (w252:refnum<vi>)
              n83 = for {
                N: w249 -> [_]
                tunnel: w255 -> [w278]
                i -> [w279]
                n84 = local read "random array main"() -> (w277:dbl[])
                n85 = Wait Until Next ms Multiple(millisecond multiple=10) -> ()  [unwired: 1 out]
                n86 = Random Number (0-1)() -> (number: 0 to 1=w281:dbl)
                n87 = Replace Array Subset(array=w277, new element=w281, index=w279) -> (w276:dbl[])
                n88 = Build Cluster Array(w278, w276) -> (→"rand plot main":cluster{i32, "element":dbl}[])
                n89 = local write "random array main"(w276) -> ()
                "cycle #" <- w279
              }
              n90 = local read "random array sub"() -> (w254:dbl[])
              n91 = control-ref of="rand plot sub"() -> (w256:refnum<vi>)
              n92 = local write "state"("subvi and real time plot" ("state")) -> ()
              n93 = call "test.vi"("length"=w249, "subvi cycle"=w250, "sample array"=w255, "rand array sub"=w254, "subvi timing"=w252, "Graph Refnum"=w256, "start time"=w251, "rand array sub refnum"=w253) -> ()  [unwired: 4 in]
              n94 = while {
                tunnel: w251 -> [w273]
                tunnel: w249 -> [w267]
                i -> [w269]
                stop <- w274 stop-if-true
                n95 = Multiply(x=w267, y=10) -> (x*y=w268:i32)
                n96 = call <vilib>:"High Resolution Relative Seconds.vi"() -> ("relative seconds"=w272:dbl)
                n97 = Greater?(x=w268, y=w269) -> (0:w274:bool)
                n98 = Subtract(x=w272, y=w273) -> (x-y=w271:dbl)
                "total\ntime" <- w271
                n99 = Divide(x=w271, y=w269) -> (x/y=→"timing average":dbl)
                n100 = Wait Until Next ms Multiple(millisecond multiple=1) -> ()  [unwired: 1 out]
                "pick-up cycle" <- w269
              }
            }
          }
        }
      }
    }
    frame Enabled {
    }
  }
  n101 = Not A Number/Path/Refnum?(number/path/refnum=w75) -> (NaN/Path/Refnum?=w17:bool)
  n102 = case shown="True" w17 {
    tunnel: [w283 w285] -> w12
    tunnel: [_ w284] -> w13
    tunnel: w75 -> [w283 _]
    frame False {
    }
    frame True {
      n103 = xnode "Open FPGA VI Reference"("resource name"=T22 "RIO0") -> ("FPGA VI Reference Out"=w285:refnum<k20>, "error out"=w284:errorcluster)  [unwired: 1 in]
    }
  }
  "fpga_reference\nOpen error out" <- w13
  n104 = disable-structure shown="Enabled" {
    disable-tunnel: w15 -> [w287 _]
    frame Enabled {
      n105 = while {
        tunnel: w287 -> [w295]
        i -> [w305]
        stop <- w306 stop-if-true
        n106 = local read "Fixed T-60sec before T1 = T0"() -> (w291:i32)
        n107 = local read "Pre-start time (ms) of DAQ \nTypically set to 1000 ms"() -> (w301:i32)
        n108 = Divide(x=w291, y=1000) -> (x/y=w289:dbl)
        n109 = Divide(x=w301, y=1000) -> (x/y=w298:dbl)
        n110 = To Quad Integer(1:w298) -> (0:w299:i64)
        n111 = To Quad Integer(1:w289) -> (0:w288:i64)
        n112 = Subtract(x=w288, y=w299) -> (x-y=w296:i64)
        n113 = call <vilib>:"High Resolution Relative Seconds.vi"() -> ("relative seconds"=w293:dbl)
        n114 = To Double Precision Float(number=w296) -> (double precision float=w297:dbl)
        n115 = Add(x=w295, y=w297) -> (x+y=w294:dbl)
        n116 = Subtract(x=w294, y=w293) -> (x-y=→"Time until Acqusition":dbl)
        n117 = Get Date/Time In Seconds() -> (seconds since 1Jan1904=w312:timestamp)
        "current epoch time timestamp" <- w312
        n118 = To Quad Integer(1:w312) -> (0:w314:i64)
        n119 = Subtract(x=w314, y=2082844800) -> (x-y=w310:i64)
        n120 = Multiply(x=1000000000, y=w310) -> (x*y=w302:i64)
        "Number of nanoseconds with offset to 1904" <- w302
        n121 = Wait Until Next ms Multiple(millisecond multiple=1) -> ()  [unwired: 1 out]
        n122 = local read "state"() -> (w307:string)
        n123 = Equal?(x="Acquiring Data...", y=w307) -> (x = y?=w306:bool)
        n124 = Equal?(x=w305, y=0) -> (x = y?=w303:bool)
        n125 = case shown="True" w303 {
          tunnel: w302 -> [_ w315]
          frame False {
          }
          frame True {
            n126 = local write "start time"(w315) -> ()
            "start time" <- w315
          }
        }
      }
    }
    frame Disabled {
    }
  }
  n127 = disable-structure shown="Enabled" {
    frame Enabled {
      n128 = case shown="False" "Read geometry from file?" {
        tunnel: [w318 w319] -> w316
        frame False {
          n129 = call "load_kbolott_volume.vi"() -> ("output"=w318:dbl[][])
        }
        frame True {
          n130 = call-poly <vilib>:"Read From Spreadsheet File.vi"("delimiter (\\t)"="" ("delimiter (\\t)"), "format (%.3f)"="%.12f", "max characters/row  (no limit:0)"=0, "number of rows (all:-1)"=-1, "file path (dialog if empty)"="Path to kbolott and volume data file") -> ("all rows"=w319:dbl[][])  [unwired: 2 in, 4 out]
        }
      }
      "kbolott_and_volume" <- w316
      n131 = local write "kbolott_and_volume"(w316) -> ()
    }
    frame Disabled {
    }
  }
  n132 = disable-structure shown="Enabled" {
    frame Enabled {
      n133 = Not(x="Read Channel Selection from file") -> (.not. x?=→"Channel Selection\nfrom input?":bool)
      n134 = case shown="True" "Read Channel Selection from file" {
        tunnel: ["channel selection input" w332] -> w328
        frame False {
        }
        frame True {
          n135 = call-poly <vilib>:"Read From Spreadsheet File.vi"("delimiter (\\t)"="\t" ("delimiter (\\t)"), "format (%d)"="%d", "max characters/row  (no limit:0)"=0, "start of read offset (chars.:0)"=0, "number of rows (all:-1)"=-1, "file path (dialog if empty)"="Path to channel selection file") -> ("all rows"=w332:i64[][])  [unwired: 1 in, 4 out]
          "file import" <- w332
        }
      }
      "final channel selection" <- w328
      n136 = Array Size(array=w328) -> (size(s)=w327:i32[])
      n137 = local write "final channel selection"(w328) -> ()
      n138 = Index Array(array=w327, index=0) -> (element=→"final channel\nselection size":i32)
    }
    frame Disabled {
    }
  }
  n139 = disable-structure shown="Enabled" {
    frame Enabled {
      n140 = Not(x="?") -> (.not. x?=w342:bool)
      "Take Input for DAC?" <- w342
      n141 = case shown="False" w342 {
        tunnel: "DAC settings file location" -> [w350 _]
        tunnel: [w344 "input DAC settings"] -> w339
        frame False {
          n142 = call-poly <vilib>:"Read From Spreadsheet File.vi"("format (%d)"="%d", "max characters/row  (no limit:0)"=58, "number of rows (all:-1)"=-1, "file path (dialog if empty)"=w350) -> ("all rows"=w345:i64[][])  [unwired: 3 in, 4 out]
          "full DAC\nfile input" <- w345
          n143 = Reshape Array(w345, 128 ("dimension size")) -> (w344:i64[])
        }
        frame True {
        }
      }
      "DAC settings" <- w339
      n144 = local write "input DAC settings"(w339) -> ()
      n145 = Array Size(array=w339) -> (size(s)=→"size(s)":i32)
      "Take file for DAC?" <- "?"
    }
    frame Disabled {
    }
  }
  n146 = flat-sequence {
    tunnel: "Cancel" ("name (unnamed)") -> [w361]
    tunnel: "Transferred1" ("name (unnamed)") -> [w360]
    tunnel: u32 0 -> [w359]
    tunnel: FALSE -> [w358]
    tunnel: [w357] -> w216
    tunnel: [w356] -> w215
    tunnel: [w355] -> w214
    tunnel: [w354] -> w213
    tunnel: [u32 0] -> w78
    frame #0 {
      n147 = local write "stop"(FALSE ("stop")) -> ()
      n148 = RT FIFO Create(0:w360, 1:w359) -> (8:w354:refnum<k33>, 11:w355:errorcluster)  [unwired: 2 in, 5 out]
      n149 = RT FIFO Create(0:w361, 1:w358) -> (8:w357:refnum<k33>, 11:w356:errorcluster)  [unwired: 3 in, 4 out]
    }
  }
  n150 = xnode "Read/Write Control"("FPGA VI Reference In"=w12, "error in"=w13, "cancel"=TRUE ("clrFifo"), "Test"=FALSE) -> ("FPGA VI Reference Out"=w225:refnum<k20>, "error out"=w224:errorcluster)
  n151 = flat-sequence {
    tunnel: w225 -> [w368]
    tunnel: w224 -> [w367]
    tunnel: [w366] -> w223
    tunnel: [w365] -> w222
    frame #0 {
      n152 = Wait (ms)(milliseconds to wait=u32 100) -> ()  [unwired: 1 out]
      n153 = xnode "Invoke Method"("FPGA VI Reference In"=w368, "error in"=w367, "IRQ Number(s)"=i32[] [0, 1, 2, 3]) -> ("FPGA VI Reference Out"=w366:refnum<k20>, "error out"=w365:errorcluster)
      "state" <- "Start (100 ms)" ("state")
    }
  }
  n154 = node-c288() -> (w208:T23)  [unwired: 1 in, 4 out]
  n155 = timed-loop {
    tunnel: w216 -> [w379]
    tunnel: w215 -> [w378]
    tunnel: w214 -> [w377]
    tunnel: w213 -> [w376]
    tunnel: [w375] -> w210
    tunnel: [w374] -> w209
    tunnel: [w373] -> w212
    tunnel: [w372] -> w211
    timing: w208 -> [_]
    timing-out: [_] -> w207
    shift-right: [w369] -> _
    shift-left: w78 -> [w370]
    stop <- "stop" stop-if-true
    n156 = RT FIFO Read(0:w376, 1:w370, 3:w377) -> (8:w373:refnum<k33>, 9:w369:u32, 11:w372:errorcluster)  [unwired: 3 out]
    n157 = RT FIFO Write(0:w379, 1:"Cancel Button", 3:w378) -> (8:w375:refnum<k33>, 11:w374:errorcluster)  [unwired: 1 in, 3 out]
    "Acquired Samples:" <- w370
  }
  n158 = flat-sequence {
    tunnel: w222 -> [w384]
    tunnel: [w383] -> w204
    tunnel: w223 -> [w385]
    tunnel: [w386] -> w186
    frame #0 {
      n159 = local write "state"("Reset" ("state")) -> ()
      n160 = call "hReset2014.vi"("error in"=w384, "FPGA VI Reference In"=w385) -> ("error out"=w383:errorcluster, "FPGA VI Reference Out"=w386:refnum<k20>)  [unwired: 4 in]
    }
  }
  n161 = node-c288(w207) -> (→"loop error":errorcluster)  [unwired: 6 out]
  n162 = call "hFilterReg2014.vi"("error in"=w204, "Filter Modus"=u16 61 ("t"), "Frequenz"=u8 79 ("AC 1kHz Frequenz\nSKIP=0"), "FPGA VI Reference In"=w186) -> ("error out"=w189:errorcluster, "Timed Out"=w198:bool, "FPGA VI Reference Out"=w188:refnum<k20>)  [unwired: 1 in]
  "FilterTimeOut" <- w198
  n163 = call "hModeReg2014.vi"("error in"=w189, "Mode"=u16 41144, "FPGA VI Reference In"=w188) -> ("error out"=w192:errorcluster, "Timeout"=w202:bool, "FPGA VI Reference Out"=w195:refnum<k20>)  [unwired: 2 in]
  n164 = call "hModeReg2014.vi"("error in"=w192, "Mode"=u16 32952, "FPGA VI Reference In"=w195) -> ("error out"=w191:errorcluster, "Timeout"=w203:bool, "FPGA VI Reference Out"=w194:refnum<k20>)  [unwired: 2 in]
  n165 = flat-sequence {
    tunnel: w212 -> [w392]
    tunnel: w211 -> [w391]
    tunnel: w210 -> [w390]
    tunnel: w209 -> [w389]
    frame #0 {
      n166 = RT FIFO Delete(0:w392, 3:w391) -> ()  [unwired: 1 in, 1 out]
      n167 = RT FIFO Delete(0:w390, 3:w389) -> ()  [unwired: 1 in, 1 out]
      n168 = local write "stop"(FALSE ("stop")) -> ()
    }
  }
  n169 = call "hModeReg2014.vi"("error in"=w191, "Mode"=u16 8376, "FPGA VI Reference In"=w194) -> ("error out"=w200:errorcluster, "Timeout"=w201:bool, "FPGA VI Reference Out"=w199:refnum<k20>)  [unwired: 2 in]
  n170 = Compound Arithmetic op=OR(w202, w203, w201, w198) -> (w187:bool)
  "result" <- w187
  n171 = case shown="False" w187 {
    tunnel: [w456 w1095] -> w73
    tunnel: [w455 w1094] -> w221
    tunnel: w199 -> [w611 w1095]
    tunnel: w200 -> [w610 w1094]
    tunnel: [w474 _] -> w1
    tunnel: [w510 _] -> w155
    tunnel: [w505 _] -> w156
    tunnel: [w501 _] -> w153
    tunnel: [w498 _] -> w154
    tunnel: [w453 _] -> w76
    tunnel: [w496 _] -> w138
    tunnel: [w495 _] -> w77
    tunnel: [w494 _] -> w137
    tunnel: [w493 _] -> w136
    tunnel: [w472 _] -> w135
    tunnel: [w476 _] -> w29
    tunnel: w16 -> [w447 _]
    tunnel: [w446 _] -> w48
    tunnel: [w414 _] -> _
    frame False {
      w516 = 2000
      w527 = u8 125  # Frequenz
      w570 = 0.0008 ("FPGSampleTime")
      w565 = 0.0
      w436 = 40.0  # Rcable
      w605 = 10.0  # Rload
      w625 = sgl 0.0004  # dt
      w626 = sgl 0.0  # tstart
      w629 = sgl 0.0004  # dt
      w630 = sgl 0.0  # tstart
      w634 = sgl 80.0 ("Scale(mV)")
      # "Offset Shift manually disabled because not need for low power discharges"
      # "Local TDMS Data Storage"
      # "Absolute Timer [ms] (Now)\n-\nAbsolute Timer [ms] (At Start)\n=\nTime need until start of DAQ"
      # "Startzeit - 14 s"
      # "old time from OP1"
      # "Store raw data"
      # "#Timing \n\nAC measurements\n2.083 kHz\nwith SKIP=1 \n\n= 5MHz/16/(3*45+15)"
      # "#Offset measurement"
      # "#Offset applied"
      # "#Range for measurements"
      # "A=> Internal full scale calibration\n8=> Internal zero scale calibration\nC=> System Zero scale Calibration\n2=> Continuous conversion\n\n2.5V reference\n80 mV scale\nChannel 2 input (voltage at shunt)\nMaster clock disable\n\np.15 7730 manual"
      n172 = flat-sequence {
        tunnel: [w762] -> w451
        tunnel: [w761] -> w450
        tunnel: w611 -> [w765]
        tunnel: w610 -> [w764]
        tunnel: w516 -> [w770]
        tunnel: [w769] -> w518
        tunnel: w451 -> [w772]
        tunnel: w450 -> [w771]
        tunnel: [w768] -> w517
        tunnel: [w786] -> w689
        tunnel: [w785] -> w688
        tunnel: [w784] -> w437
        tunnel: w516 -> [w782]
        tunnel: w518 -> [w779]
        tunnel: w517 -> [w780]
        frame #0 {
          n173 = call "Wait3"("Count(mSec)"=u32 3000) -> ()  [unwired: 1 out]
          n174 = call "hComRegStart2013.vi"("error in"=w764, "FPGA VI Reference In"=w765) -> ("error out"=w761:errorcluster, "Timed Out"=→"Timed Out 2":bool, "FPGA VI Reference Out"=w762:refnum<k20>)  [unwired: 3 in]
        }
        frame #1 {
          n175 = local write "state"("SyncRun (1000 ms)" ("state")) -> ()
          n176 = call "Wait6"("Count(mSec)"=u32 1000) -> ()  [unwired: 1 out]
          n177 = call "hSync&StartSampling2013.vi"("error in"=w771, "#Samples"=w770, "FPGA VI Reference In"=w772) -> ("error out"=w769:errorcluster, "FPGA VI Reference Out"=w768:refnum<k20>)  [unwired: 1 in]
        }
        frame #2 {
          n178 = xnode "Read/Write Control"("FPGA VI Reference In"=w780, "error in"=w779, "ScanID"=u32 1) -> ("FPGA VI Reference Out"=w775:refnum<k20>, "error out"=w774:errorcluster)
          n179 = xnode "Read/Write Control"("FPGA VI Reference In"=w775, "error in"=w774) -> ("FPGA VI Reference Out"=w781:refnum<k20>, "error out"=w778:errorcluster, "ScanID"=→"ScanID 2":u32)
          "ScandID read/write error, early" <- w778
          n180 = call "hReadChannelsRTDMA2013.vi"("FPGA VI Reference In"=w781, "Nsamples"=w782, "error in"=w778) -> ("FPGA VI Reference Out"=w786:refnum<k20>, "Fehler"=→"Fehler":bool, "RawArray"=w784:i16[][], "error out"=w785:errorcluster)  [unwired: 2 in]
          "error after hReadDMA" <- w785
          n181 = local write "state"("ReadOffset" ("state")) -> ()
        }
      }
      n182 = property on="Acquired Samples:" class="Slide (strict)"("Scale.Range:Maximum"=w516) -> ()  [unwired: 2 in, 2 out]
      n183 = call "hSoftReset2013.vi"("error in"=w688, "FPGA VI Reference In"=w689) -> ("error out"=w525:errorcluster, "FPGA VI Reference Out"=w520:refnum<k20>)  [unwired: 4 in]
      n184 = call "Int2Volt2D.vi"("IntegerArray"=w437, "Scale(mV)"=sgl 80.0) -> ("RealArray"=w561:sgl[][])
      n185 = xnode "Read/Write Control"("FPGA VI Reference In"=w520, "error in"=w525, "HIREF"=TRUE) -> ("FPGA VI Reference Out"=w523:refnum<k20>, "error out"=w522:errorcluster)
      n186 = for {
        tunnel: w561 -> [w807] mode=indexing
        tunnel: [w806] -> w558 mode=indexing
        tunnel: [w805] -> w560 mode=indexing
        tunnel: [w804] -> w559 mode=indexing
        n187 = Array Subset(array=w807, index=500, length=1000) -> (w809:sgl[])
        n188 = Array Max & Min(array=w809) -> (max value=w812:sgl, min value=w813:sgl)  [unwired: 2 out]
        n189 = Subtract(x=w812, y=w813) -> (x-y=w806:sgl)
        n190 = call <vilib>:"Std Deviation and Variance.vi"("X"=w809, "Weighting (Sample)"=enum16{"Sample", "Population"}."Population") -> ("mean"=w805:dbl, "standard deviation"=w804:dbl)  [unwired: 1 out]
      }
      "Offset (V)" <- w560
      n191 = call "hFilterReg2014.vi"("error in"=w522, "Filter Modus"=u16 512 ("t"), "Frequenz"=w527, "FPGA VI Reference In"=w523) -> ("error out"=w521:errorcluster, "FPGA VI Reference Out"=w524:refnum<k20>)  [unwired: 1 in, 1 out]
      n192 = Array Subset(array=w561, index (row)=0, length (row)=64, index (col)=0) -> (w575:sgl[][])  [unwired: 1 in]
      n193 = Array Subset(array=w561, index (row)=64, length (row)=64, index (col)=0) -> (w571:sgl[][])  [unwired: 1 in]
      n194 = call "hModeReg2014.vi"("error in"=w521, "Mode"=u16 41017, "FPGA VI Reference In"=w524) -> ("error out"=w531:errorcluster, "FPGA VI Reference Out"=w530:refnum<k20>)  [unwired: 2 in, 1 out]
      n195 = call "Visualize_Signals64.vi"("FPGSampleTime"=w570, "tstart"=w565, "Signals"=w575) -> ("plot(Signals) 33-64"=→"Offset 33-64":T26, "plot(Signals) 1-32"=→"Offset 1-32":T4)  [unwired: 7 in]
      n196 = call "Visualize_Signals64.vi"("FPGSampleTime"=w570, "tstart"=w565, "Signals"=w571) -> ("plot(Signals) 33-64"=→"Offset 97 - 128":T26, "plot(Signals) 1-32"=→"Offset 65 - 96":T4)  [unwired: 7 in]
      n197 = call "hModeReg2014.vi"("error in"=w531, "Mode"=u16 32825, "FPGA VI Reference In"=w530) -> ("error out"=w528:errorcluster, "FPGA VI Reference Out"=w529:refnum<k20>)  [unwired: 2 in, 1 out]
      n198 = call "hModeReg2014.vi"("error in"=w528, "Mode"=u16 8249, "FPGA VI Reference In"=w529) -> ("error out"=w421:errorcluster, "FPGA VI Reference Out"=w422:refnum<k20>)  [unwired: 2 in, 1 out]
      n199 = disable-structure shown="Enabled" {
        disable-tunnel: w422 -> [w699 w705]
        disable-tunnel: w421 -> [w698 w704]
        disable-tunnel: [w697 w705] -> w420
        disable-tunnel: [w696 w704] -> w419
        frame Disabled {
          n200 = xnode "Read/Write Control"("FPGA VI Reference In"=w699, "error in"=w698, "ScanID"=u32 1) -> ("FPGA VI Reference Out"=w701:refnum<k20>, "error out"=w700:errorcluster)
          n201 = xnode "Read/Write Control"("FPGA VI Reference In"=w701, "error in"=w700) -> ("FPGA VI Reference Out"=w697:refnum<k20>, "error out"=w696:errorcluster, "ScanID"=→"ScanID":u32)
          "ScandID read/write error, late" <- w696
        }
        frame Enabled {
        }
      }
      n202 = Multiply(x=w559, y=1000000.0 ("Scale")) -> (x*y=→"StandardDeviation\n        (microV)":dbl[])
      n203 = Multiply(x=w558, y=1000000.0 ("Scale")) -> (x*y=→"Peak to Peak \n      (microV)":dbl[])
      n204 = Multiply(x=w560, y=1000.0 ("Scale")) -> (x*y=w476:dbl[])
      "Mean (mV)" <- w476
      n205 = control-ref of="Cancel Button"() -> (w686:refnum<vi>)
      n206 = control-ref of="Acquired Samples:"() -> (w684:refnum<vi>)
      n207 = control-ref of="state"() -> (w685:refnum<vi>)
      n208 = call "hCalRT2013.vi"("FPGA VI Reference In"=w420, "cancelbutton"=w686, "state"=w685, "Acquired Samples"=w684, "error in"=w419) -> ("FPGA VI Reference Out"=w608:refnum<k20>, "Ref"=w633:i16[][], "Meas"=w682:i16[][], "error out"=w607:errorcluster)  [unwired: 6 in, 1 out]
      "error out Cal" <- w607
      n209 = call "Int2Volt2D.vi"("IntegerArray"=w633, "Scale(mV)"=w634) -> ("RealArray"=w635:sgl[][])
      n210 = call "Int2Volt2D.vi"("IntegerArray"=w682, "Scale(mV)"=w634) -> ("RealArray"=w683:sgl[][])
      n211 = flat-sequence {
        tunnel: w608 -> [w797]
        tunnel: w607 -> [w795]
        tunnel: [w796] -> w536
        tunnel: [w794] -> w535
        tunnel: [w801] -> w491
        tunnel: [w800] -> w564
        tunnel: w536 -> [w803]
        tunnel: w535 -> [w802]
        frame #0 {
          w791 = FALSE ("RESET")
          n212 = call "Wait"("Count(mSec)"=u16 3000 ("Count(uSec)")) -> ()  [unwired: 1 out]
          n213 = xnode "Read/Write Control"("FPGA VI Reference In"=w797, "error in"=w795, "RLY1"=w791, "RLY2"=w791, "HIREF"=w791, "Sprung0"=w791, "Sprung1"=w791, "ScanID"=u32 0, "Test"="Switch to fixed \nCalibration Values", "RESET"=TRUE) -> ("FPGA VI Reference Out"=w796:refnum<k20>, "error out"=w794:errorcluster)
          n214 = local write "state"("SoftReset (3000 ms)" ("state")) -> ()
        }
        frame #1 {
          n215 = xnode "Read/Write Control"("FPGA VI Reference In"=w803, "error in"=w802, "RESET"=FALSE) -> ("FPGA VI Reference Out"=w800:refnum<k20>, "error out"=w801:errorcluster)
          n216 = call "Wait5"("Count(mSec)"=u16 1000 ("Count(uSec)")) -> ()  [unwired: 1 out]
        }
      }
      n217 = case shown="True" "SecondFilter" {
        tunnel: [w742 w751] -> w446
        tunnel: [w741 w749] -> w515
        tunnel: [w740 w750] -> w514
        frame False {
          # "#Timing \n\nAC measurements\n2.5 kHz\nwith SKIP=1 \n\n= 5MHz/16/(3*37+14)"
          n218 = disable-structure shown="Enabled" {
            disable-tunnel: [u16 574 ("t") u16 575 ("t")] -> w740
            disable-tunnel: [u16 37 ("frequenz") u16 45 ("frequenz")] -> w741
            disable-tunnel: [sgl 0.0004 sgl 0.00048] -> w742
            frame Enabled {
            }
            frame Disabled {
            }
          }
        }
        frame True {
          # "#Timing \n\nAC measurements\n1.25 kHz\nwith SKIP=0 \n\n= 5MHz/16/250"
          n219 = call "FreqSel.vi"("Ring"="FreqSelRing") -> ("Frequency"=w749:u16, "DLY"=w750:u16, "SampleTime"=w751:sgl)  [unwired: 1 out]
        }
      }
      "SampleTime" <- w446
      n220 = xnode "Invoke Method"("FPGA VI Reference In"=w564, "error in"=w491, "Requested Depth"=u32 256) -> ("FPGA VI Reference Out"=w492:refnum<k20>, "error out"=w490:errorcluster, "Actual Depth"=→"Actual Depth":u32)
      n221 = call "hFilterReg2014.vi"("error in"=w490, "Filter Modus"=w514, "Frequenz"=w515, "FPGA VI Reference In"=w492) -> ("error out"=w624:errorcluster, "FPGA VI Reference Out"=w623:refnum<k20>)  [unwired: 1 in, 1 out]
      n222 = local read "input DAC settings"() -> (w445:i64[])
      "RangeIndex" <- w445
      n223 = case shown="False" "global or individual DAC settings for knob" {
        tunnel: w624 -> [w1063 w1079]
        tunnel: w623 -> [w1064 w1078]
        tunnel: [w1058 w1077] -> w562
        tunnel: [w1061 w1069] -> w563
        tunnel: u16 41096 -> [w1056 w1068]
        tunnel: u16 49288 -> [_ w1070]
        tunnel: u16 8328 -> [w1057 w1066]
        tunnel: w445 -> [w1055 _]
        tunnel: u16 32904 -> [w1053 w1067]
        frame False {
          # "MIddle Previously connected xC088 not to x8088"
          n224 = call "hModeRegRange2013.vi"("error in"=w1063, "RangeArray"=w1055, "Mode"=w1056, "FPGA VI Reference In"=w1064) -> ("error out"=w1060:errorcluster, "FPGA VI Reference Out"=w1062:refnum<k20>)  [unwired: 1 in, 1 out]
          n225 = call "hModeRegRange2013.vi"("error in"=w1060, "RangeArray"=w1055, "Mode"=w1053, "FPGA VI Reference In"=w1062) -> ("error out"=w1059:errorcluster, "FPGA VI Reference Out"=w1054:refnum<k20>)  [unwired: 1 in, 1 out]
          n226 = call "hModeRegRange2013.vi"("error in"=w1059, "RangeArray"=w1055, "Mode"=w1057, "FPGA VI Reference In"=w1054) -> ("error out"=w1058:errorcluster, "FPGA VI Reference Out"=w1061:refnum<k20>)  [unwired: 1 in, 1 out]
        }
        frame True {
          n227 = call "hModeReg2014.vi"("error in"=w1079, "Range"="DAC Range Setting", "Mode"=w1068, "FPGA VI Reference In"=w1078) -> ("error out"=w1075:errorcluster, "FPGA VI Reference Out"=w1076:refnum<k20>)  [unwired: 1 in, 1 out]
          n228 = call "hModeReg2014.vi"("error in"=w1075, "Range"="DAC Range Setting", "Mode"=w1067, "FPGA VI Reference In"=w1076) -> ("error out"=w1073:errorcluster, "FPGA VI Reference Out"=w1074:refnum<k20>)  [unwired: 1 in, 1 out]
          n229 = disable-structure shown="Enabled" {
            disable-tunnel: w1074 -> [w1085 w1087]
            disable-tunnel: w1073 -> [w1084 w1086]
            disable-tunnel: [w1083 w1087] -> w1072
            disable-tunnel: [w1082 w1086] -> w1071
            disable-tunnel: w1070 -> [w1081 _]
            disable-tunnel: "DAC Range Setting" -> [w1080 _]
            frame Disabled {
              n230 = call "hModeReg2014.vi"("error in"=w1084, "Range"=w1080, "Mode"=w1081, "FPGA VI Reference In"=w1085) -> ("error out"=w1082:errorcluster, "FPGA VI Reference Out"=w1083:refnum<k20>)  [unwired: 1 in, 1 out]
            }
            frame Enabled {
            }
          }
          n231 = call "hModeReg2014.vi"("error in"=w1071, "Range"="DAC Range Setting", "Mode"=w1066, "FPGA VI Reference In"=w1072) -> ("error out"=w1077:errorcluster, "FPGA VI Reference Out"=w1069:refnum<k20>)  [unwired: 1 in, 1 out]
        }
      }
      n232 = flat-sequence {
        tunnel: w484 -> [w820]
        tunnel: w538 -> [w822]
        tunnel: [w821] -> w487
        tunnel: [w819] -> w486
        tunnel: [w817] -> w443
        tunnel: [w816] -> w442
        tunnel: [w815] -> w407
        tunnel: [w814] -> w406
        tunnel: w487 -> [w871]
        tunnel: [w871] -> w481
        tunnel: w486 -> [w870]
        tunnel: [w870] -> w479
        tunnel: w447 -> [w860]
        tunnel: w443 -> [w858]
        tunnel: w442 -> [w857]
        tunnel: [w853] -> w413
        tunnel: [w852] -> w410
        tunnel: w407 -> [w839]
        tunnel: w406 -> [w838]
        tunnel: [w835] -> w404
        tunnel: [w834] -> w402
        tunnel: w481 -> [w937]
        tunnel: [w936] -> w480
        tunnel: w479 -> [w935]
        tunnel: [w934] -> w478
        tunnel: w429 -> [w933]
        tunnel: w413 -> [w932]
        tunnel: [w932] -> w412
        tunnel: w410 -> [w931]
        tunnel: [w931] -> w409
        tunnel: [w930] -> w405
        tunnel: w404 -> [w930]
        tunnel: [w929] -> w403
        tunnel: w402 -> [w929]
        tunnel: w480 -> [w942]
        tunnel: w478 -> [w943]
        tunnel: w447 -> [w944]
        tunnel: [w942] -> w469
        tunnel: [w943] -> w468
        tunnel: w412 -> [w941]
        tunnel: [w941] -> w411
        tunnel: w409 -> [w940]
        tunnel: [w940] -> w408
        tunnel: w405 -> [w939]
        tunnel: w403 -> [w938]
        tunnel: [w939] -> w400
        tunnel: [w938] -> w398
        tunnel: w469 -> [w954]
        tunnel: w468 -> [w953]
        tunnel: [w954] -> w467
        tunnel: [w953] -> w466
        tunnel: [w952] -> w465
        tunnel: [w951] -> w441
        tunnel: [w950] -> w440
        tunnel: w411 -> [w951]
        tunnel: w408 -> [w950]
        tunnel: [w949] -> w401
        tunnel: w400 -> [w949]
        tunnel: [w948] -> w399
        tunnel: w398 -> [w948]
        tunnel: w467 -> [w971]
        tunnel: w466 -> [w972]
        tunnel: w465 -> [w969]
        tunnel: w429 -> [w963]
        tunnel: w418 -> [w970]
        tunnel: [w968] -> w463
        tunnel: [w969] -> w462
        tunnel: [w967] -> w461
        tunnel: [w966] -> w460
        tunnel: [w965] -> w459
        tunnel: [w964] -> w458
        tunnel: w441 -> [w962]
        tunnel: w440 -> [w961]
        tunnel: [w960] -> w439
        tunnel: [w959] -> w438
        tunnel: w401 -> [w958]
        tunnel: w399 -> [w957]
        tunnel: [w956] -> w397
        tunnel: [w955] -> w396
        tunnel: [w1049] -> w455
        tunnel: [w1050] -> w393
        tunnel: [w1046] -> w415
        tunnel: [w1051] -> w456
        tunnel: [w1052] -> w444
        tunnel: w462 -> [w1052]
        tunnel: w461 -> [w1051]
        tunnel: w460 -> [w1046]
        tunnel: w459 -> [w1050]
        tunnel: w458 -> [w1049]
        tunnel: [w1047] -> w457
        tunnel: w439 -> [w1045]
        tunnel: w438 -> [w1044]
        tunnel: [w1045] -> w431
        tunnel: [w1044] -> w430
        tunnel: w397 -> [w1043]
        tunnel: w396 -> [w1042]
        tunnel: [w1043] -> w395
        tunnel: [w1042] -> w394
        frame #0 {
          n233 = disable-structure shown="Enabled" {
            disable-tunnel: [w825 _] -> w815
            disable-tunnel: [w824 _] -> w814
            frame Enabled {
              # "channel preselection for output AO"
              n234 = call-poly <vilib>:"DAQmx Create Virtual Channel.vi"("maximum value"="maximum voltage @ 10MW single channel", "minimum value"=0.0, "physical channels"="DAQmx Physical Channel\nsingle channel") -> ("task out"=w825:refnum<k21>, "error out"=w824:errorcluster)  [unwired: 11 in]
            }
            frame Disabled {
            }
          }
          n235 = disable-structure shown="Enabled" {
            disable-tunnel: [w830 _] -> w817
            disable-tunnel: [w829 _] -> w816
            frame Enabled {
              # "channel preselection for output AO"
              n236 = call-poly <vilib>:"DAQmx Create Virtual Channel.vi"("maximum value"="maximum voltage @ 10MW\nP_rad estimate", "minimum value"=0.0, "physical channels"="DAQmx Physical Channel\nP_rad estimate") -> ("task out"=w830:refnum<k21>, "error out"=w829:errorcluster)  [unwired: 11 in]
            }
            frame Disabled {
            }
          }
          n237 = call "hComRegStart2013.vi"("error in"=w820, "FPGA VI Reference In"=w822) -> ("error out"=w819:errorcluster, "FPGA VI Reference Out"=w821:refnum<k20>)  [unwired: 3 in, 1 out]
          n238 = local write "state"("Calibration Done" ("state")) -> ()
          n239 = call "Wait4"("Count(mSec)"=u32 1000) -> ()  [unwired: 1 out]
        }
        frame #1 {
          (unwired) 15000  # fixed -15sec for T0
          n240 = local read "Switch to fixed \nCalibration Values"() -> (w851:bool)
          n241 = case shown="True" w851 {
            tunnel: [w874 w876] -> w850
            tunnel: [w873 w877] -> w856
            tunnel: [w872 w875] -> w849
            frame False {
              n242 = local read "KappaM"() -> (w874:dbl[])
              n243 = local read "RMESS"() -> (w873:dbl[])
              n244 = local read "TauM"() -> (w872:dbl[])
            }
            frame True {
              n245 = local read "Kappa00"() -> (w876:dbl[])
              n246 = local read "Tau00"() -> (w875:dbl[])
              n247 = local read "RB000"() -> (w877:dbl[])
            }
          }
          n248 = disable-structure shown="Enabled" {
            frame Enabled {
              # "pre-allocation of the sample and signal arrays from the subroutine of measurement"
              # "make sample array that is used in the real time P_rad plot"
              n249 = local read "No. of Samples\n[TOA / Sample Rate]"() -> (w921:u32)
              n250 = Initialize Array(0, w921) -> (w918:i32[])
              "Nsample array" <- w918
              n251 = Initialize Array(0.0, w921) -> (w920:dbl[])
              n252 = local write "Nsample array"(w918) -> ()
              n253 = local write "final P_rad"(w920) -> ()
              n254 = local write "av power array"(w920) -> ()
              n255 = for {
                N: w921 -> [_]
                i -> [w923]
                n256 = local read "Nsample array"() -> (w924:i32[])
                n257 = Replace Array Subset(array=w924, new element=w923, index=w923) -> (w922:i32[])
                n258 = local write "Nsample array"(w922) -> ()
              }
            }
            frame Disabled {
            }
          }
          n259 = Subtract(x="Fixed T-60sec before T1 = T0", y="Pre-start time (ms) of DAQ \nTypically set to 1000 ms") -> (x-y=w863:i32)
          "Total wait time (TWT)\nTypically 59 s" <- w863
          n260 = disable-structure shown="Enabled" {
            disable-tunnel: w858 -> [w914 _]
            disable-tunnel: w857 -> [w913 _]
            disable-tunnel: [w912 _] -> w855
            disable-tunnel: [w911 _] -> w854
            disable-tunnel: w839 -> [w908 _]
            disable-tunnel: w838 -> [w907 _]
            disable-tunnel: [w903 _] -> w837
            disable-tunnel: [w902 _] -> w836
            frame Enabled {
              # "sampling rate and mode to continuous"
              # "sampling rate and mode to continuous"
              n261 = property class="DAQmx Write"(reference=w914, error in=w913, "RegenMode"="RegenMode") -> (reference out=w916:refnum<k21>, error out=w915:errorcluster)
              n262 = property class="DAQmx Write"(reference=w908, error in=w907, "RegenMode"="RegenMode") -> (reference out=w910:refnum<k21>, error out=w909:errorcluster)
              n263 = call-poly <vilib>:"DAQmx Timing.vi"("task/channels in"=w916, "sample mode"="sample mode", "rate"="rate of voltage sampling", "error in"=w915) -> ("task out"=w912:refnum<k21>, "error out"=w911:errorcluster)  [unwired: 10 in]
              n264 = call-poly <vilib>:"DAQmx Timing.vi"("task/channels in"=w910, "sample mode"="sample mode", "rate"="rate of voltage sampling", "error in"=w909) -> ("task out"=w903:refnum<k21>, "error out"=w902:errorcluster)  [unwired: 10 in]
            }
            frame Disabled {
            }
          }
          n265 = Add(x=w860, y=w863) -> (x+y=w861:u32)
          n266 = call "power_factors.vi"("TauM"=w849, "KappaM"=w850, "RMESS"=w856) -> ("F_ch"=w847:dbl[], "tau_fact"=w848:dbl[])  [unwired: 7 in]
          "F_ch" <- w847
          "tau_fact" <- w848
          n267 = Tick Count (ms)() -> (millisecond timer value=w865:u32)
          n268 = local read "kbolott_and_volume"() -> (w846:dbl[][])
          n269 = local read "SampleTime"() -> (w845:sgl)
          n270 = local read "Offset (V)"() -> (w844:dbl[])
          n271 = Subtract(x=w861, y=w865) -> (x-y=w866:u32)
          "Calibration Time" <- w866
          n272 = Subtract(x=w866, y=u32 50) -> (x-y=w867:u32)
          "Countdown Time" <- w867
          n273 = Add(x=w865, y=w867) -> (x+y=w868:u32)
          n274 = while {
            tunnel: w868 -> [w927]
            stop <- w928 continue-if-true
            n275 = Tick Count (ms)() -> (millisecond timer value=w926:u32)
            n276 = Subtract(x=w927, y=w926) -> (x-y=w925:u32)
            "DAQ Timer" <- w925
            n277 = Greater?(x=w927, y=w926) -> (0:w928:bool)
            n278 = local write "DAQ Timer"(w925) -> ()
          }
          n279 = disable-structure shown="Enabled" {
            disable-tunnel: w855 -> [w891 _]
            disable-tunnel: w854 -> [w890 _]
            disable-tunnel: [w889 _] -> w853
            disable-tunnel: [w888 _] -> w852
            disable-tunnel: w837 -> [w884 _]
            disable-tunnel: w836 -> [w883 _]
            disable-tunnel: [w879 _] -> w835
            disable-tunnel: [w878 _] -> w834
            frame Enabled {
              # "channel prepartions with larger array for busyness"
              # "number of samples to write until renewal"
              # "rate of sampling"
              # "5 milliseconds"
              n280 = local read "rate of voltage sampling"() -> (w900:dbl)
              n281 = Multiply(x=0.005, y=w900) -> (x*y=w896:dbl)
              n282 = local read "maximum voltage @ 10MW\nP_rad estimate"() -> (w887:dbl)
              n283 = Round To Nearest(number=w896) -> (nearest integer value=w894:dbl)
              "number of samples per iteration" <- w894
              n284 = Multiply(x=w894, y=2.0) -> (x*y=w893:dbl)
              n285 = Initialize Array(0.0 ("element"), w893) -> (w880:dbl[])
              "empty write array" <- w880
              n286 = call-poly <vilib>:"DAQmx Write.vi"("task/channels in"=w884, "data"=w880, "error in"=w883) -> ("task out"=w882:refnum<k21>, "error out"=w881:errorcluster)  [unwired: 10 in, 1 out]
              n287 = call-poly <vilib>:"DAQmx Write.vi"("task/channels in"=w891, "data"=w880, "error in"=w890) -> ("task out"=w899:refnum<k21>, "number of samples written per channel"=→"number of samples written on channel":u32, "error out"=w898:errorcluster)  [unwired: 10 in]
              n288 = Divide(x=10.0, y=w887) -> (x/y=→"nominator":dbl)
              n289 = call <vilib>:"DAQmx Start Task.vi"("task/channels in"=w899, "error in"=w898) -> ("task out"=w889:refnum<k21>, "error out"=w888:errorcluster)  [unwired: 12 in]
              n290 = call <vilib>:"DAQmx Start Task.vi"("task/channels in"=w882, "error in"=w881) -> ("task out"=w879:refnum<k21>, "error out"=w878:errorcluster)  [unwired: 12 in]
            }
            frame Disabled {
            }
          }
          n291 = call "calculate_Ud_estimate.vi"("Tau_ch"=w849, "kbolott_and_volume"=w846, "Kappa_ch"=w850, "F_ch"=w847, "SampleTime"=w845, "tau_fact"=w848, "estimated floating voltage"="estimated floating voltage", "Offset (V)"=w844, "elected channel for output"="selected channel for output via second analog channel") -> ("voltage factor"=→"voltage factor":dbl, "estimated voltage"=→"estimated voltage @ 10 MW":dbl)  [unwired: 9 in]
          n292 = local write "state"("Countdown Timer" ("state")) -> ()
        }
        frame #2 {
          # "takes 50 ms"
          n293 = call "hSync&StartSampling2013.vi"("error in"=w935, "#Samples"=w933, "FPGA VI Reference In"=w937) -> ("error out"=w934:errorcluster, "FPGA VI Reference Out"=w936:refnum<k20>)  [unwired: 1 in]
        }
        frame #3 {
          n294 = Tick Count (ms)() -> (millisecond timer value=w945:u32)
          n295 = local write "state"("SyncRun" ("state")) -> ()
          n296 = Subtract(x=w945, y=w944) -> (x-y=→"DAQ wait time (should be = TWT":u32)
        }
        frame #4 {
          n297 = call "Tick Count"() -> ("Tick Count(mSec)"=w952:u32)
        }
        frame #5 {
          n298 = disable-structure shown="Enabled" {
            disable-tunnel: w962 -> [w978 _]
            disable-tunnel: w961 -> [w981 _]
            disable-tunnel: [w980 _] -> w960
            disable-tunnel: [w979 _] -> w959
            disable-tunnel: w958 -> [w977 _]
            disable-tunnel: w957 -> [w976 _]
            disable-tunnel: [w975 _] -> w956
            disable-tunnel: [w974 _] -> w955
            frame Enabled {
              # "voltage loop until halt and empty channel to 0 V"
              n299 = while {
                tunnel: w981 -> [w1007]
                tunnel: [w1005] -> w979
                tunnel: w978 -> [w1008]
                tunnel: [w1006] -> w980
                tunnel: w977 -> [w993]
                tunnel: w976 -> [w992]
                tunnel: [w991] -> w975
                tunnel: [w990] -> w974
                stop <- w1003 stop-if-true
                # "actually writing smaller data"
                n300 = disable-structure shown="Enabled" {
                  frame Enabled {
                    n301 = local read "single channel voltage array"() -> (w1009:dbl[])
                    n302 = local read "av power array"() -> (w1012:dbl[])
                    n303 = local read "Nsample array"() -> (w1011:i32[])
                    n304 = Build Cluster Array(w1011, w1012, w1009) -> (→"real time P_rad plot":cluster{i32, "element":dbl, "element":dbl}[])
                  }
                  frame Disabled {
                  }
                }
                n305 = local read "current P_rad sample [MW]"() -> (w996:dbl)
                n306 = local read "current single channel voltage"() -> (w985:dbl)
                n307 = local read "nominator"() -> (w995:dbl)
                n308 = local read "No. of Samples\n[TOA / Sample Rate]"() -> (w999:u32)
                n309 = local read "number of samples per iteration"() -> (w987:dbl)
                n310 = local read "Acquired Samples:"() -> (w1000:u32)
                n311 = Multiply(x=w985, y="voltage fac") -> (x*y=w982:dbl)
                n312 = Divide(x=w996, y=w995) -> (x/y=w983:dbl)
                n313 = Initialize Array(w983, w987) -> (w994:dbl[])
                n314 = Initialize Array(w982, w987) -> (w986:dbl[])
                n315 = call-poly <vilib>:"DAQmx Write.vi"("task/channels in"=w1008, "data"=w994, "error in"=w1007) -> ("task out"=w1006:refnum<k21>, "number of samples written per channel"=→"number of samples \nwritten per channel":u32, "error out"=w1005:errorcluster)  [unwired: 10 in]
                n316 = local write "single channel voltage output [MW]"(w982) -> ()
                n317 = call-poly <vilib>:"DAQmx Write.vi"("task/channels in"=w993, "data"=w986, "error in"=w992) -> ("task out"=w991:refnum<k21>, "error out"=w990:errorcluster)  [unwired: 10 in, 1 out]
                n318 = local write "P_rad output\nvoltage"(w983) -> ()
                n319 = Unbundle(w990) -> ("status"=w989:bool, "source"=→"single channel output error source":string)  [unwired: 1 out]
                n320 = Greater Or Equal?(x=w1000, y=w999) -> (x >= y?=w998:bool)
                n321 = Unbundle(w1005) -> ("status"=w1004:bool, "source"=→"P_rad analog output error source":string)  [unwired: 1 out]
                n322 = Compound Arithmetic op=OR(w1004, "Stop Voltage Output", w998, w989) -> (w1003:bool)
              }
            }
            frame Disabled {
            }
          }
          n323 = disable-structure shown="Enabled" {
            disable-tunnel: w972 -> [w1033 w1040]
            disable-tunnel: w971 -> [w1032 w1041]
            disable-tunnel: w963 -> [w1031 w1039]
            disable-tunnel: [w1030 w1038] -> w967
            disable-tunnel: [w1029 w1037] -> w964
            disable-tunnel: [w1028 _] -> w968
            disable-tunnel: [w1025 _] -> w966
            disable-tunnel: [w1027 w1035] -> w965
            disable-tunnel: w970 -> [w1026 _]
            frame Enabled {
              n324 = local read "selected channel for output via second analog channel"() -> (w1014:i32)
              n325 = local read "tau_fact"() -> (w1019:dbl[])
              n326 = control-ref of="current single channel voltage"() -> (w1015:refnum<vi>)
              n327 = local read "F_ch"() -> (w1018:dbl[])
              n328 = local read "kbolott_and_volume"() -> (w1021:dbl[][])
              n329 = local read "final channel selection"() -> (w1024:i64[][])
              n330 = local read "SampleTime"() -> (w1020:sgl)
              n331 = control-ref of="av power array"() -> (w1023:refnum<vi>)
              n332 = control-ref of="current P_rad sample [MW]"() -> (w1022:refnum<vi>)
              n333 = local read "Offset (V)"() -> (w1016:dbl[])
              n334 = control-ref of="single channel voltage array"() -> (w1013:refnum<vi>)
              n335 = local read "Tau"() -> (w1017:dbl[])
              n336 = call "hReadChannels-UandP-2018.vi"("FPGA VI Reference In"=w1032, "SampleTime"=w1020, "final channel selection"=w1024, "kbolott_and_volume"=w1021, "Nsamples"=w1031, "tau_channels"=w1017, "error in"=w1033, "F_Ch"=w1018, "Scale(mV)"=w1026, "Offset (V)"=w1016, "av power array"=w1023, "single channel number"=w1014, "single channel voltage"=w1015, "voltage array"=w1013, "tau_fact"=w1019, "current P_rad sample"=w1022) -> ("Fehler"=w1028:bool, "FPGA VI Reference Out"=w1030:refnum<k20>, "PowerArray"=w1025:sgl[][], "RawArray"=w1027:sgl[][], "error out"=w1029:errorcluster)  [unwired: 7 in]
            }
            frame Disabled {
              n337 = call "hReadChannelsRTDMA2013.vi"("FPGA VI Reference In"=w1041, "Nsamples"=w1039, "error in"=w1040) -> ("FPGA VI Reference Out"=w1038:refnum<k20>, "RawArray"=w1036:i16[][], "error out"=w1037:errorcluster)  [unwired: 2 in, 1 out]
              n338 = call "Int2Volt2D.vi"("IntegerArray"=w1036, "Scale(mV)"=sgl 80.0) -> ("RealArray"=w1035:sgl[][])
            }
          }
          n339 = local write "state"("Acquiring Data..." ("state")) -> ()
        }
        frame #6 {
          n340 = local write "state"("Acquiring done" ("state")) -> ()
          n341 = call "Tick Count2"() -> ("Tick Count(mSec)"=w1047:u32)
        }
      }
      n342 = disable-structure shown="Enabled" {
        disable-tunnel: w563 -> [w758 w759]
        disable-tunnel: w562 -> [w757 w760]
        disable-tunnel: w445 -> [w756 _]
        disable-tunnel: [w755 _] -> w542
        disable-tunnel: [w754 w759] -> w538
        disable-tunnel: [w753 w760] -> w485
        frame Disabled {
          n343 = call "hDACsubtract2013.vi"("FPGA VI Reference In"=w758, "Ranges"=w756, "error in"=w757) -> ("FPGA VI Reference Out"=w754:refnum<k20>, "DACbits"=w755:u16[], "error out"=w753:errorcluster)  [unwired: 10 in]
        }
        frame Enabled {
        }
      }
      n344 = local read "SampleTime"() -> (w427:sgl)
      n345 = Divide(x="Time of Acqusition [s]", y=w427) -> (x/y=w434:dbl)
      n346 = Round To Nearest(number=w434) -> (nearest integer value=w433:dbl)
      n347 = To Unsigned Long Integer(number=w433) -> (unsigned 32bit integer=w429:u32)
      "No. of Samples\n[TOA / Sample Rate]" <- w429
      n348 = property on="Acquired Samples:" class="Slide (strict)"(error in=w485, "Scale.Range:Maximum"=w429) -> (error out=w484:errorcluster)  [unwired: 1 in, 1 out]
      "sampling error" <- w484
      n349 = Subtract(x=w542, y=u16 1024 ("NSample")) -> (x-y=→"DACbits 2":u16[])
      n350 = To Double Precision Float(number=w429) -> (double precision float=w428:dbl)
      n351 = Multiply(x=w428, y=w427) -> (x*y=w426:dbl)
      n352 = Multiply(x=w426, y=1000.0) -> (x*y=→"predicted time [ms] to finalize DAQ":dbl)
      n353 = Divide(x=w683, y=w605) -> (x/y=w502:dbl[][])
      n354 = call "CalFaktor-128.vi"("CalCurrent(t)"=w502, "Rload"=w605, "Rcable"=w436) -> ("FitData"=w497:dbl[][], "Kappa"=w453:dbl[], "Tau"=w495:dbl[], "RB01"=w496:dbl[])  [unwired: 1 out]
      "KappaM" <- w453
      n355 = Array Subset(array=w502, index (row)=0 ("index"), length (row)=128 ("length")) -> (w501:dbl[][])  [unwired: 2 in]
      n356 = Add(x=w436, y=w605) -> (x+y=w604:dbl)
      n357 = Multiply(x=w604, y=2.0) -> (x*y=w602:dbl)
      n358 = local read "Switch to fixed \nCalibration Values"() -> (w622:bool)
      n359 = call "Cal(SubVI)-2013.vi"("Array"=w502, "dt"=w629, "StartChan"=64 ("ChanStart"), "tstart"=w630, "FitData"=w497) -> ("plot(Signals) 1-32"=→"MessCal 65 - 80":T27, "plot(Signals) 33-64"=→"MessCal 81 - 96":T28)  [unwired: 9 in]
      n360 = call "Cal(SubVI)-2013.vi"("Array"=w502, "dt"=w629, "StartChan"=96 ("ChanStart"), "tstart"=w630, "FitData"=w497) -> ("plot(Signals) 1-32"=→"MessCal 97 - 112":T27, "plot(Signals) 33-64"=→"MessCal 113 - 128":T28)  [unwired: 9 in]
      n361 = call "Cal(SubVI)-2013.vi"("Array"=w502, "dt"=w629, "StartChan"=32 ("ChanStart"), "tstart"=w630, "FitData"=w497) -> ("plot(Signals) 1-32"=→"MessCal 33 - 49":T27, "plot(Signals) 33-64"=→"MessCal 49 - 64":T28)  [unwired: 9 in]
      n362 = call "Cal(SubVI)-2013.vi"("Array"=w502, "dt"=w629, "StartChan"=0 ("ChanStart"), "tstart"=w630, "FitData"=w497) -> ("plot(Signals) 1-32"=→"MessCal 1-16":T27, "plot(Signals) 33-64"=→"MessCal 17-32":T28)  [unwired: 9 in]
      n363 = call "Arraylimit128.vi"("LowerLimit"=2e-05, "Array Input"=w453, "UpperLimit"=0.002) -> ("BoolArray"=w676:bool[])  [unwired: 1 out]
      n364 = call "Arraylimit128.vi"("LowerLimit"=400.0, "Array Input"=w496, "UpperLimit"=2000.0) -> ("BoolArray"=w674:bool[], "ArrayOutput"=w452:dbl[])
      "RMESS" <- w452
      n365 = call "Arraylimit128.vi"("LowerLimit"=0.001, "Array Input"=w495, "UpperLimit"=0.8) -> ("BoolArray"=w675:bool[], "ArrayOutput"=w454:dbl[])
      "TauM" <- w454
      n366 = case shown="True" w622 {
        tunnel: [w1089 "RB000"] -> w606
        tunnel: [w1088 "Kappa00"] -> w601
        tunnel: [w1090 "Tau00"] -> w464
        tunnel: w495 -> [w1090 _]
        tunnel: w496 -> [w1089 _]
        tunnel: w453 -> [w1088 _]
        frame False {
        }
        frame True {
        }
      }
      n367 = disable-structure shown="Enabled" {
        disable-tunnel: w606 -> [w695 _]
        disable-tunnel: w602 -> [w694 _]
        disable-tunnel: w601 -> [w693 _]
        disable-tunnel: w464 -> [w692 _]
        frame Enabled {
          n368 = call "U2PCoeff.vi"("Numeric"=w694, "Kappa00"=w693, "RB000"=w695) -> ("Array"=→"ScalPower":dbl[], "Array 2"=→"RawScal":dbl[])
          "Tau" <- w692
        }
        frame Disabled {
        }
      }
      n369 = disable-structure shown="Enabled" {
        disable-tunnel: w415 -> [w713 _]
        disable-tunnel: w393 -> [w709 _]
        frame Enabled {
          n370 = local read "No. of Samples\n[TOA / Sample Rate]"() -> (w715:u32)
          n371 = local read "kbolott_and_volume"() -> (w714:dbl[][])
          n372 = call "rawpower2totalprad.vi"("PowerArray [W]"=w713, "No. of Samples\n[TOA / Sample Rate]"=w715, "kbolott_and_volume"=w714) -> ("full P_rad [MW]"=w711:dbl[])
          "final P_rad" <- w711
          n373 = local read "voltage fac"() -> (w707:dbl)
          n374 = local read "single channel voltage array"() -> (w708:dbl[])
          n375 = Multiply(x=w707, y=w708) -> (x*y=w706:dbl[])
          n376 = local read "Nsample array"() -> (w712:i32[])
          n377 = Build Cluster Array(w712, w706, w711) -> (w710:cluster{i32, dbl, "element":dbl}[])
          n378 = local write "real time P_rad plot"(w710) -> ()
          "PowerArray" <- w713
          "RawArray" <- w709
        }
        frame Disabled {
        }
      }
      n379 = disable-structure shown="Enabled" {
        disable-tunnel: w431 -> [w726 _]
        disable-tunnel: w430 -> [w725 _]
        disable-tunnel: w395 -> [w722 _]
        disable-tunnel: w394 -> [w721 _]
        frame Enabled {
          w719 = u16 0 items=["OK message + warnings"]
          w727 = u16 0 items=["OK message + warnings"]
          # "place empty channel values and free resources"
          n380 = local read "empty write array"() -> (w720:dbl[])
          n381 = call-poly <vilib>:"DAQmx Write.vi"("task/channels in"=w722, "data"=w720, "error in"=w721) -> ("task out"=w723:refnum<k21>, "error out"=w724:errorcluster)  [unwired: 10 in, 1 out]
          n382 = call-poly <vilib>:"DAQmx Write.vi"("task/channels in"=w726, "data"=w720, "error in"=w725) -> ("task out"=w728:refnum<k21>, "error out"=w729:errorcluster)  [unwired: 10 in, 1 out]
          n383 = call <vilib>:"DAQmx Clear Task.vi"("task in"=w723, "error in"=w724) -> ("error out"=w718:errorcluster)  [unwired: 13 in]
          n384 = call <vilib>:"DAQmx Clear Task.vi"("task in"=w728, "error in"=w729) -> ("error out"=w717:errorcluster)  [unwired: 13 in]
          n385 = Bundle("error out"=w717, "error out"=w718) -> (→"voltage sampling error":T17)  [unwired: 1 in]
          n386 = call <vilib>:"Simple Error Handler.vi"("type of dialog (OK msg:1)"=w719, "error in (no error)"=w718) -> ()  [unwired: 3 in, 5 out]
          n387 = call <vilib>:"Simple Error Handler.vi"("type of dialog (OK msg:1)"=w727, "error in (no error)"=w717) -> ()  [unwired: 3 in, 5 out]
        }
        frame Disabled {
        }
      }
      n388 = Scale By Power Of 2(n=w445, x=sgl 10.0 ("Scale(mV)")) -> (x*2^n=w418:sgl[])
      "x*2^n" <- w418
      n389 = Compound Arithmetic op=OR(w676, w675, w674) -> (w659:bool[])
      n390 = local read "Pre-start time (ms) of DAQ \nTypically set to 1000 ms"() -> (w483:i32)
      n391 = Array Subset(array=w659, index=0, length=32) -> (→"MessStatus 1-32":bool[])
      n392 = Array Subset(array=w659, index=32, length=32) -> (→"MessStatus 33-64":bool[])
      n393 = Array Subset(array=w659, index=64, length=32) -> (→"MessStatus 65-96":bool[])
      n394 = Array Subset(array=w659, index=96, length=32) -> (→"MessStatus 97-128":bool[])
      n395 = Divide(x=w635, y=w605) -> (x/y=w511:dbl[][])
      n396 = Divide(x=w483, y=sgl -1000.0 ("Scale(mV)")) -> (x/y=w449:sgl)
      "T-Start [for Display)\nShould be -1 [s]" <- w449
      n397 = call "CalFaktor-128.vi"("CalCurrent(t)"=w511, "Rload"=w605, "Rcable"=w436) -> ("FitData"=w448:dbl[][], "Kappa"=w472:dbl[], "Tau"=w493:dbl[], "RB01"=w494:dbl[])  [unwired: 1 out]
      "KappaR" <- w472
      n398 = Array Subset(array=w511, index (row)=0 ("index"), length (row)=128 ("length")) -> (w510:dbl[][])  [unwired: 2 in]
      n399 = call "Cal(SubVI)-2013.vi"("Array"=w511, "dt"=w625, "StartChan"=0 ("ChanStart"), "tstart"=w626, "FitData"=w448) -> ("plot(Signals) 1-32"=→"RefCal 1-16":T27, "plot(Signals) 33-64"=→"RefCal 17-32":T28)  [unwired: 9 in]
      n400 = call "Cal(SubVI)-2013.vi"("Array"=w511, "dt"=w625, "StartChan"=32 ("ChanStart"), "tstart"=w626, "FitData"=w448) -> ("plot(Signals) 1-32"=→"RefCal 33 - 48":T27, "plot(Signals) 33-64"=→"RefCal 49 - 64":T28)  [unwired: 9 in]
      n401 = call "Cal(SubVI)-2013.vi"("Array"=w511, "dt"=w625, "StartChan"=64 ("ChanStart"), "tstart"=w626, "FitData"=w448) -> ("plot(Signals) 1-32"=→"RefCal 65 - 80":T27, "plot(Signals) 33-64"=→"RefCal 81 - 96":T28)  [unwired: 9 in]
      n402 = call "Cal(SubVI)-2013.vi"("Array"=w511, "dt"=w625, "StartChan"=96 ("ChanStart"), "tstart"=w626, "FitData"=w448) -> ("plot(Signals) 1-32"=→"RefCal 97 - 112":T27, "plot(Signals) 33-64"=→"RefCal 113 - 128":T28)  [unwired: 9 in]
      n403 = Array Subset(array=w448, index (row)=0 ("index"), length (row)=128 ("length")) -> (w505:dbl[][])  [unwired: 2 in]
      n404 = call "Arraylimit128.vi"("LowerLimit"=400.0, "Array Input"=w494, "UpperLimit"=2000.0) -> ("BoolArray"=w644:bool[], "ArrayOutput"=w471:dbl[])
      "RREF" <- w471
      n405 = call "Arraylimit128.vi"("LowerLimit"=2e-05, "Array Input"=w472, "UpperLimit"=0.002) -> ("BoolArray"=w642:bool[])  [unwired: 1 out]
      n406 = call "Arraylimit128.vi"("LowerLimit"=0.001, "Array Input"=w493, "UpperLimit"=0.8) -> ("BoolArray"=w643:bool[], "ArrayOutput"=w473:dbl[])
      "TauR" <- w473
      n407 = Subtract(x=w457, y=w444) -> (x-y=→"Measured Time for DAQ [ms]\n\nApprox. ~ SampleTime * Samples":u32)
      n408 = Compound Arithmetic op=OR(w642, w643, w644) -> (w423:bool[])
      n409 = Array Subset(array=w415, index (row)=64, length (row)=64, index (col)=0) -> (w591:sgl[][])  [unwired: 1 in]
      n410 = Array Subset(array=w415, index (row)=0, length (row)=64, index (col)=0) -> (w595:sgl[][])  [unwired: 1 in]
      n411 = Array Subset(array=w393, index (row)=64, length (row)=64, index (col)=0) -> (w475:sgl[][])  [unwired: 1 in]
      n412 = Array Subset(array=w393, index (row)=0, length (row)=64, index (col)=0) -> (w470:sgl[][])  [unwired: 1 in]
      n413 = Array Subset(array=w393, index (row)=0 ("index"), length (row)=128 ("length")) -> (w474:sgl[][])  [unwired: 2 in]
      n414 = Array Subset(array=w415, index (row)=0 ("index"), length (row)=128 ("length")) -> (w414:sgl[][])  [unwired: 2 in]
      n415 = Array Subset(array=w423, index=0, length=32) -> (→"RefStatus 1-32":bool[])
      n416 = Array Subset(array=w423, index=32, length=32) -> (→"RefStatus 33-64":bool[])
      n417 = Array Subset(array=w423, index=64, length=32) -> (→"RefStatus 65-96":bool[])
      n418 = Array Subset(array=w423, index=96, length=32) -> (→"RefStatus 97-128":bool[])
      n419 = disable-structure shown="Enabled" {
        disable-tunnel: w393 -> [w739 _]
        disable-tunnel: w473 -> [w738 _]
        disable-tunnel: w472 -> [w737 _]
        disable-tunnel: w471 -> [w736 _]
        disable-tunnel: w470 -> [w735 _]
        disable-tunnel: w454 -> [w734 _]
        disable-tunnel: w453 -> [w733 _]
        disable-tunnel: w452 -> [w732 _]
        disable-tunnel: w449 -> [w731 _]
        disable-tunnel: w446 -> [w730 _]
        frame Disabled {
          n420 = call "W7-X-Bolo-TMDS-LOCAL.vi"("Kappa 2"=w737, "ArrayOutput 4"=w738, "ArrayOutput 3"=w736, "Array"=w735, "RawArray"=w739, "Numeric"=w731, "ArrayOutput"=w732, "Kappa"=w733, "ArrayOutput 2"=w734, "SampleTime"=w730) -> ()  [unwired: 5 in, 1 out]
        }
        frame Enabled {
        }
      }
      n421 = call "Visualize_Signals64.vi"("FPGSampleTime"=w446, "tstart"=w449, "Signals"=w591) -> ("plot(Signals) 33-64"=→"Pow 97 - 128":T26, "plot(Signals) 1-32"=→"Pow 65 - 96":T4)  [unwired: 7 in]
      n422 = call "Visualize_Signals64.vi"("FPGSampleTime"=w446, "tstart"=w449, "Signals"=w595) -> ("plot(Signals) 33-64"=→"Pow 33-64":T26, "plot(Signals) 1-32"=→"Pow 1-32":T4)  [unwired: 7 in]
      n423 = call "Visualize_Signals64.vi"("FPGSampleTime"=w446, "tstart"=w449, "Signals"=w475) -> ("plot(Signals) 33-64"=→"Raw 97 - 128":T26, "plot(Signals) 1-32"=→"Raw 65 - 97":T4)  [unwired: 7 in]
      n424 = call "Visualize_Signals64.vi"("FPGSampleTime"=w446, "tstart"=w449, "Signals"=w470) -> ("plot(Signals) 33-64"=→"Raw 33-64":T26, "plot(Signals) 1-32"=→"Raw 1-32":T4)  [unwired: 7 in]
      n425 = Array Subset(array=w497, index (row)=0 ("index"), length (row)=128 ("length")) -> (w498:dbl[][])  [unwired: 2 in]
      "Fehler READ U+P" <- w463
    }
    frame True {
      n426 = local write "state"("Error->NoRead" ("state")) -> ()
    }
  }
  n427 = xnode "Read/Write Control"("FPGA VI Reference In"=w73) -> ("FPGA VI Reference Out"=w46:refnum<k20>, "SampleTrigger2"=w74:u32)  [unwired: 1 in, 1 out]
  n428 = Multiply(x=w48, y=w47) -> (x*y=w26:i64)
  n429 = To Quad Integer(1:w74) -> (0:w42:i64)
  "Presamples \n(If -1, then no trigger detected)" <- w42
  n430 = flat-sequence {
    tunnel: w17 -> [w1100]
    tunnel: w221 -> [w1101]
    tunnel: w46 -> [w1102]
    tunnel: [w1102] -> w45
    tunnel: [w1101] -> w44
    tunnel: [w1100] -> w43
    tunnel: w26 -> [w1099]
    tunnel: w42 -> [w1098]
    tunnel: [w1097] -> w41
    tunnel: [w1115] -> w40
    tunnel: [w1114] -> w39
    tunnel: [w1113] -> w38
    tunnel: w45 -> [w1115]
    tunnel: w44 -> [w1114]
    tunnel: w43 -> [w1113]
    tunnel: w40 -> [w1122]
    tunnel: [w1122] -> w36
    tunnel: w39 -> [w1121]
    tunnel: [w1121] -> w34
    tunnel: w38 -> [w1120]
    tunnel: [w1120] -> w32
    tunnel: [w1118] -> w37
    tunnel: w36 -> [w1130]
    tunnel: [w1130] -> w35
    tunnel: w34 -> [w1129]
    tunnel: [w1129] -> w33
    tunnel: w32 -> [w1128]
    tunnel: [w1128] -> w31
    tunnel: w35 -> [w1136]
    tunnel: w33 -> [w1134]
    tunnel: w31 -> [w1133]
    frame #0 {
      n431 = case "Correct timebase depending on if Trigger detected" shown="4294967295" w1098 {
        selector: w1098 -> [w1105 _]
        tunnel: [w1106 w1108] -> w1097
        tunnel: w1099 -> [w1104 _]
        frame Default {
          # "1 Trigger nur während OP"
          # "4294967295"
          # "Trigger deviation [ns]"
          # "Input Sample Frequency"
          n432 = Multiply(x=w1105, y=w1104) -> (x*y=w1103:i64)
          n433 = To Quad Integer(1:w1103) -> (0:w1106:i64)
        }
        frame 4294967295 {
          # "ms to ns conversion"
          # "4294967295\n=default if not Trigger"
          n434 = local read "DAQ wait time (should be = TWT"() -> (w1107:i32)
          n435 = Multiply(x=i64 1000000, y=w1107) -> (x*y=w1108:i64)
        }
      }
    }
    frame #1 {
      n436 = control-ref of="DAQ Timer"() -> (w1110:refnum<vi>)
      n437 = call "W7X-Bolo-Timer.vi"("Wait-Time until Trigger\npublished on CODA\ntypically 10 s"="waiting time 'til trigger\npublished by CODAC", "Digital in"=w1110) -> ()  [unwired: 10 in]
      n438 = local write "state"("Wait for published Shot Time (10s)" ("state")) -> ()
    }
    frame #2 {
      n439 = case shown="3" "Trigger Source" {
        tunnel: [w1123 w1125 "Set Manual Time [ns], default updated last on 06/20/2018" w1127] -> w1118
        tunnel: "Trigger No Choice\nfrom MDS+ Website\n0 for old\n1 during OP" -> [_ w1124 _ _]
        frame 0 {
          n440 = call "Get UTC from NTP.vi"() -> ("UTC Time"=w1123:i64)  [unwired: 10 in, 1 out]
        }
        frame 1, Default {
          n441 = call "GetTriggerTime.vi"("TriggerIndex (1)"=w1124) -> ("TriggerTime [ns]"=w1125:i64)  [unwired: 9 in, 1 out]
        }
        frame 2 {
        }
        frame 3 {
          n442 = local read "start time"() -> (w1127:i64)
        }
      }
      n443 = local write "state"("Reading Trigger Time" ("state")) -> ()
    }
    frame #3 {
    }
    frame #4 {
      n444 = case shown="True" w1133 {
        tunnel: w1136 -> [w1137 w1139]
        tunnel: w1134 -> [_ w1138]
        tunnel: [w1137 _] -> w1132
        frame False {
        }
        frame True {
          n445 = xnode "Close FPGA VI Reference"("FPGA VI Reference In"=w1139, "error in"=w1138) -> ()  [unwired: 1 out]
        }
      }
      "FPGA VI Reference Out" <- w1132
      n446 = local write "state"("Idle / Waiting for new Trigger" ("state")) -> ()
      n447 = property on="stop" class="Bool (strict)"("Val(Sgnl)"=TRUE) -> ()  [unwired: 2 in, 2 out]
    }
  }
  n448 = call "Array_Trans.vi"("RB01"=w137, "Array 8"=w29, "Kappa 2"=w135, "RB01 2"=w138, "Tau 2"=w136, "Kappa"=w76, "Tau"=w77) -> ("Array 7"=w131:dbl[][], "Array 4"=w126:dbl[][], "Array"=w121:dbl[][], "Array 3"=w124:dbl[][], "Array 6"=w130:dbl[][], "Array 2"=w122:dbl[][], "Array 5"=w128:dbl[][])  [unwired: 2 in]
  n449 = Multiply(x=w26, y=w28) -> (x*y=w27:i64)
  n450 = local read "No. of Samples\n[TOA / Sample Rate]"() -> (w30:u32)
  n451 = Add(x=w37, y=w41) -> (x+y=w55:i64)
  n452 = To Quad Integer(1:w55) -> (0:w181:i64)
  n453 = Build Array(w55) -> (w79:i64[])
  n454 = call "W7X2DJSON.vi"("values"=w131, "label"=w105, "dimensionSize"=w53, "dimensions"=w79, "dimensionCount"=128, "sampleCount"=w53, "datatype"=w133) -> ("JSON string"=w104:string)  [unwired: 4 in]
  n455 = call "W7X2DJSON.vi"("values"=w121, "label"=w86, "dimensionSize"=w84, "dimensions"=w79, "dimensionCount"=128, "sampleCount"=w84, "datatype"=w149) -> ("JSON string"=w85:string)  [unwired: 4 in]
  n456 = call "W7X2DJSON.vi"("values"=w130, "label"=w102, "dimensionSize"=w82, "dimensions"=w79, "dimensionCount"=128, "sampleCount"=w82, "datatype"=w139) -> ("JSON string"=w101:string)  [unwired: 4 in]
  n457 = call "W7X2DJSON.vi"("values"=w128, "label"=w99, "dimensionSize"=w127, "dimensions"=w79, "dimensionCount"=128, "sampleCount"=w127, "datatype"=w141) -> ("JSON string"=w98:string)  [unwired: 4 in]
  n458 = Initialize Array(w55, w30) -> (w151:i64[])
  n459 = for {
    N: w30 -> [_]
    shift-right: [w1144] -> w71
    shift-left: w151 -> [w1145]
    shift-right: [w1141] -> _
    shift-left: w55 -> [w1142]
    tunnel: w27 -> [w1140]
    i -> [w1143]
    n460 = Add(x=w1142, y=w1140) -> (x+y=w1141:i64)
    n461 = Replace Array Subset(array=w1145, new element=w1142, index=w1143) -> (w1144:i64[])
  }
  n462 = call "W7X2DJSON.vi"("values"=w126, "label"=w96, "dimensionSize"=w125, "dimensions"=w79, "dimensionCount"=128, "sampleCount"=w125, "datatype"=w143) -> ("JSON string"=w95:string)  [unwired: 4 in]
  n463 = call "W7X2DJSON.vi"("values"=w124, "label"=w93, "dimensionSize"=w123, "dimensions"=w79, "dimensionCount"=128, "sampleCount"=w123, "datatype"=w145) -> ("JSON string"=w92:string)  [unwired: 4 in]
  n464 = call "W7X2DJSON.vi"("values"=w122, "label"=w89, "dimensionSize"=w83, "dimensions"=w79, "dimensionCount"=128, "sampleCount"=w83, "datatype"=w147) -> ("JSON string"=w88:string)  [unwired: 4 in]
  n465 = Initialize Array(w37, w54) -> (w150:i64[])
  n466 = for {
    N: w54 -> [_]
    shift-right: [w1150] -> w68
    shift-left: w150 -> [w1151]
    shift-right: [w1147] -> _
    shift-left: w55 -> [w1148]
    tunnel: w27 -> [w1146]
    i -> [w1149]
    n467 = Add(x=w1148, y=w1146) -> (x+y=w1147:i64)
    n468 = Replace Array Subset(array=w1151, new element=w1148, index=w1149) -> (w1150:i64[])
  }
  n469 = local read "SampleTime"() -> (w52:sgl)
  n470 = local read "SampleTime"() -> (w19:sgl)
  n471 = Reciprocal(x=w52) -> (1/x=w64:sgl)
  n472 = Reciprocal(x=w52) -> (1/x=w62:sgl)
  n473 = Reciprocal(x=w52) -> (1/x=w60:sgl)
  n474 = Reciprocal(x=w19) -> (1/x=w56:sgl)
  n475 = Reciprocal(x=w19) -> (1/x=w58:sgl)
  n476 = To Unsigned Word Integer(number=w56) -> (unsigned 16bit integer=w21:u16)
  n477 = To Unsigned Word Integer(number=w58) -> (unsigned 16bit integer=w57:u16)
  n478 = call "W7X2DJSON.vi"("values"=w156, "label"=w23, "dimensionSize"=w163, "dimensions"=w68, "dimensionCount"=128, "sampleCount"=w163, "datatype"=w165) -> ("JSON string"=w22:string)  [unwired: 4 in]
  n479 = call "W7X2DJSON.vi"("values"=w153, "label"=w114, "dimensionSize"=w160, "dimensions"=w68, "dimensionCount"=128, "sampleCount"=w160, "datatype"=w162) -> ("JSON string"=w113:string)  [unwired: 4 in]
  n480 = call "W7X2DJSON.vi"("values"=w155, "label"=w110, "dimensionSize"=w166, "dimensions"=w68, "dimensionCount"=128, "sampleCount"=w166, "datatype"=w168) -> ("JSON string"=w109:string)  [unwired: 4 in]
  n481 = call "W7X2DJSON.vi"("values"=w154, "label"=w120, "dimensionSize"=w157, "dimensions"=w68, "dimensionCount"=128, "sampleCount"=w157, "datatype"=w159) -> ("JSON string"=w119:string)  [unwired: 4 in]
  n482 = call "W7X2DJSON.vi"("values"=w1, "label"=w107, "dimensionSize"=w30, "dimensions"=w71, "dimensionCount"=128, "sampleCount"=w30, "datatype"=w169) -> ("JSON string"=w106:string)  [unwired: 4 in]
  n483 = To Unsigned Word Integer(number=w64) -> (unsigned 16bit integer=w63:u16)
  n484 = To Unsigned Word Integer(number=w62) -> (unsigned 16bit integer=w61:u16)
  n485 = To Unsigned Word Integer(number=w60) -> (unsigned 16bit integer=w59:u16)
  n486 = Multiply(x=w30, y=w52) -> (x*y=w51:sgl)
  n487 = Replace Array Subset(array=i64[] [1399090569999999999, -1] ("dimensions"), new element=w181, index=0) -> (w18:i64[])
  n488 = call "W7X1DPut.vi"("dimensions"=w18, "Unit"=w103, "SigJSONbuffer"=w104, "SigLabel"=w105) -> ("Parlog error out"=→"offset parlog error":errorcluster)  [unwired: 7 in]
  n489 = call "W7X1DPut.vi"("dimensions"=w18, "Unit"=w87, "SigJSONbuffer"=w85, "SigLabel"=w86) -> ("Parlog error out"=→"mTau parlog error":errorcluster)  [unwired: 7 in]
  n490 = call "W7X1DPut.vi"("dimensions"=w18, "Unit"=w100, "SigJSONbuffer"=w101, "SigLabel"=w102) -> ("Parlog error out"=→"rKappa parlog error":errorcluster)  [unwired: 7 in]
  n491 = call "W7X1DPut.vi"("dimensions"=w18, "Unit"=w97, "SigJSONbuffer"=w98, "SigLabel"=w99) -> ("Parlog error out"=→"rRes parlog error":errorcluster)  [unwired: 7 in]
  n492 = call "W7X1DPut.vi"("dimensions"=w18, "Unit"=w94, "SigJSONbuffer"=w95, "SigLabel"=w96) -> ("Parlog error out"=→"rTau parlog error":errorcluster)  [unwired: 7 in]
  n493 = call "W7X1DPut.vi"("dimensions"=w18, "Unit"=w91, "SigJSONbuffer"=w92, "SigLabel"=w93) -> ("Parlog error out"=→"mKappa parlog error":errorcluster)  [unwired: 7 in]
  n494 = call "W7X1DPut.vi"("dimensions"=w18, "Unit"=w90, "SigJSONbuffer"=w88, "SigLabel"=w89) -> ("Parlog error out"=→"mRes parlog error":errorcluster)  [unwired: 7 in]
  n495 = call "W7X2DPut.vi"("dimensions"=w18, "pulse_length"=w51, "Unit"=w108, "sample period"=w52, "sample rate"=w59, "SigJSONbuffer"=w106, "SigLabel"=w107) -> ("Parlog error out"=→"BoloSignal data error":errorcluster)  [unwired: 4 in]
  n496 = call "W7X2DPut.vi"("dimensions"=w18, "pulse_length"=4.0, "Unit"=w112, "sample period"=w52, "sample rate"=w63, "SigJSONbuffer"=w109, "SigLabel"=w110) -> ("Parlog error out"=→"BoloCalibMeasFoilCurrent\ndata error":errorcluster)  [unwired: 4 in]
  n497 = call "W7X2DPut.vi"("dimensions"=w18, "pulse_length"=4.0, "Unit"=w118, "sample period"=w19, "sample rate"=w61, "SigJSONbuffer"=w119, "SigLabel"=w120) -> ("Parlog error out"=→"BoloCalibRefFoilFit data error":errorcluster)  [unwired: 4 in]
  n498 = call "W7X2DPut.vi"("dimensions"=w18, "pulse_length"=4.0, "Unit"=w116, "sample period"=w19, "sample rate"=w57, "SigJSONbuffer"=w113, "SigLabel"=w114) -> ("Parlog error out"=→"BoloCalibRefFoilCurrent data error":errorcluster)  [unwired: 4 in]
  n499 = call "W7X2DPut_DAZ.vi"("dimensions"=w18, "pulse_length"=4.0, "Unit"=w24, "sample period"=w19, "sample rate"=w21, "SigJSONbuffer"=w22, "SigLabel"=w23) -> ("Parlog error out"=→"BoloCalibMeasFoilFit data error":errorcluster)  [unwired: 4 in]
  n500 = call "chanDescQSB.vi"("dimensions"=w18, "values"=T19 [{"chanDescs"=[{"name"="E_Chan_1", "active"=1}, {"name"="E_Chan_2", "active"=1}, {"name"="E_Chan_3", "active"=1}, {"name"="E_Chan_4", "active"=1}, {"name"="E_Chan_5", "active"=1}, {"name"="E_Chan_6", "active"=1}, {"name"="E_Chan_7", "active"=1}, {"name"="E_Chan_8", "active"=1}, {"name"="E_Chan_9", "active"=1}, {"name"="E_Chan_10", "active"=1}, {"name"="E_Chan_11", "active"=1}, {"name"="E_Chan_12", "active"=1}, {"name"="E_Chan_13", "active"=1}, {"name"="E_Chan_14", "active"=1}, {"name"="E_Chan_15", "active"=1}, {"name"="E_Chan_16", "active"=1}, {"name"="E_Chan_17", "active"=1}, {"name"="E_Chan_18", "active"=1}, {"name"="E_Chan_19", "active"=1}, {"name"="E_Chan_20", "active"=1}, {"name"="E_Chan_21", "active"=1}, {"name"="E_Chan_22", "active"=1}, {"name"="E_Chan_23", "active"=1}, {"name"="E_Chan_24", "active"=1}, {"name"="E_Chan_25", "active"=1}, {"name"="E_Chan_26", "active"=1}, {"name"="E_Chan_27", "active"=1}, {"name"="E_Chan_28", "active"=1}, {"name"="E_Chan_29", "active"=1}, {"name"="E_Chan_30", "active"=1}, {"name"="E_Chan_31", "active"=1}, {"name"="E_Chan_32", "active"=1}, {"name"="E_Chan_33", "active"=1}, {"name"="E_Chan_34", "active"=1}, {"name"="E_Chan_35", "active"=1}, {"name"="E_Chan_36", "active"=1}, {"name"="E_Chan_37", "active"=1}, {"name"="E_Chan_38", "active"=1}, {"name"="E_Chan_39", "active"=1}, {"name"="E_Chan_40", "active"=1}, {"name"="E_Chan_41", "active"=1}, {"name"="E_Chan_42", "active"=1}, {"name"="E_Chan_43", "active"=1}, {"name"="E_Chan_44", "active"=1}, {"name"="E_Chan_45", "active"=1}, {"name"="E_Chan_46", "active"=1}, {"name"="E_Chan_47", "active"=1}, {"name"="E_Chan_48", "active"=1}, {"name"="E_Chan_49", "active"=1}, {"name"="E_Chan_50", "active"=1}, {"name"="E_Chan_51", "active"=1}, {"name"="E_Chan_52", "active"=1}, {"name"="E_Chan_53", "active"=1}, {"name"="E_Chan_54", "active"=1}, {"name"="E_Chan_55", "active"=1}, {"name"="E_Chan_56", "active"=1}, {"name"="E_Chan_57", "active"=1}, {"name"="E_Chan_58", "active"=1}, {"name"="E_Chan_59", "active"=1}, {"name"="E_Chan_60", "active"=1}, {"name"="E_Chan_61", "active"=1}, {"name"="E_Chan_62", "active"=1}, {"name"="E_Chan_63", "active"=1}, {"name"="E_Chan_64", "active"=1}, {"name"="E_Chan_65", "active"=1}, {"name"="E_Chan_66", "active"=1}, {"name"="E_Chan_67", "active"=1}, {"name"="E_Chan_68", "active"=1}, {"name"="E_Chan_69", "active"=1}, {"name"="E_Chan_70", "active"=1}, {"name"="E_Chan_71", "active"=1}, {"name"="E_Chan_72", "active"=1}, {"name"="E_Chan_73", "active"=1}, {"name"="E_Chan_74", "active"=1}, {"name"="E_Chan_75", "active"=1}, {"name"="E_Chan_76", "active"=1}, {"name"="E_Chan_77", "active"=1}, {"name"="E_Chan_78", "active"=1}, {"name"="E_Chan_79", "active"=1}, {"name"="E_Chan_80", "active"=1}, {"name"="E_Chan_81", "active"=1}, {"name"="E_Chan_82", "active"=1}, {"name"="E_Chan_83", "active"=1}, {"name"="E_Chan_84", "active"=1}, {"name"="E_Chan_85", "active"=1}, {"name"="E_Chan_86", "active"=1}, {"name"="E_Chan_87", "active"=1}, {"name"="E_Chan_88", "active"=1}, {"name"="E_Chan_89", "active"=1}, {"name"="E_Chan_90", "active"=1}, {"name"="E_Chan_91", "active"=1}, {"name"="E_Chan_92", "active"=1}, {"name"="E_Chan_93", "active"=1}, {"name"="E_Chan_94", "active"=1}, {"name"="E_Chan_95", "active"=1}, {"name"="E_Chan_96", "active"=1}, {"name"="E_Chan_97", "active"=1}, {"name"="E_Chan_98", "active"=1}, {"name"="E_Chan_99", "active"=1}, {"name"="E_Chan_100", "active"=1}, {"name"="E_Chan_101", "active"=1}, {"name"="E_Chan_102", "active"=1}, {"name"="E_Chan_103", "active"=1}, {"name"="E_Chan_104", "active"=1}, {"name"="E_Chan_105", "active"=1}, {"name"="E_Chan_106", "active"=1}, {"name"="E_Chan_107", "active"=1}, {"name"="E_Chan_108", "active"=1}, {"name"="E_Chan_109", "active"=1}, {"name"="E_Chan_110", "active"=1}, {"name"="E_Chan_111", "active"=1}, {"name"="E_Chan_112", "active"=1}, {"name"="E_Chan_113", "active"=1}, {"name"="E_Chan_114", "active"=1}, {"name"="E_Chan_115", "active"=1}, {"name"="E_Chan_116", "active"=1}, {"name"="E_Chan_117", "active"=1}, {"name"="E_Chan_118", "active"=1}, {"name"="E_Chan_119", "active"=1}, {"name"="E_Chan_120", "active"=1}, {"name"="E_Chan_121", "active"=1}, {"name"="E_Chan_122", "active"=1}, {"name"="E_Chan_123", "active"=1}, {"name"="E_Chan_124", "active"=1}, {"name"="E_Chan_125", "active"=1}, {"name"="E_Chan_126", "active"=1}, {"name"="E_Chan_127", "active"=1}, {"name"="E_Chan_128", "active"=1}]}], "label"="parms") -> ()  [unwired: 1 out]
  n501 = call "parmsQSB.vi"("dimensions"=w18, "values"=T18 [{"Nchannel"=128, "ADCbits"=16, "BridgeVoltage (V)"=5.0, "ExptSampleFrequency (Hz)"=2500.0, "CalibSampleFrequency (Hz)"=2500.0, "CalStep1 (V)"="2.5", "CalStep2 (V)"="3.7", "detector"="Au_Kapton"}], "label"="parms") -> ("JSON string"=w70:string)
  n502 = call <vilib>:"OpenHandle.vi"() -> ("client handle out"=w178:T29, "error out"=w177:errorcluster)  [unwired: 14 in]
  n503 = call <vilib>:"AddHeader.vi"("client handle"=w178, "header"="Content-Type", "value"="application/json", "error in (no error)"=w177) -> ("client handle out"=w176:T29, "error out"=w175:errorcluster)  [unwired: 10 in]
  n504 = call-poly <vilib>:"POST.vi"("client handle"=w176, "url"="http://archive-webapi/Test/raw/W7X/QSB_Bolometry/File_PARLOG/", "buffer"=w70, "error in (no error)"=w175, "timeout (10000)"=400000 ("timeout for upload")) -> ("client handle out"=w180:T29, "headers"=→"headers chanDesc":string, "body"=→"body chanDesc":string, "error out"=w65:errorcluster)  [unwired: 7 in]
  n505 = call <vilib>:"CloseHandle.vi"("client handle"=w180, "error in (no error)"=w65) -> ("error out"=w170:errorcluster)  [unwired: 13 in]
  n506 = call "saveToFile.vi"("SigJSONbuffer"=w70, "dimensions"=w68, "String"="File_PARLOG" ("name or relative path")) -> ("error out"=w66:errorcluster)  [unwired: 8 in]
  n507 = Merge Errors(w170, w66) -> (→"parms error out":errorcluster)
  "trigger time final" <- w37
